vi "PH_Sequencer.panel.vi"() -> ()   [LabVIEW 2014, in "PH_Sequencer.lvlib"]
uses:
  PH_Sequencer.lvlib
  PH_Basics/PH_StatusHandler/PH_StatusHandler.GUI element.ctl
  PH_Timing/PH_Timing.Slow Trigger Settings.ctl
  PH_Timing/PH_Timing.Timing Mode.ctl
  PH_Timing/PH_Timing.Phase FEs.ctl
  PH_Sequencer.PU Information for GUI.ctl
  PH_Basics/PH_PowerUnit_BaseClass/PH_PowerUnit_BaseClass.SM States.ctl
  PH_Beamline_Chief/PH_Beamline_Chief.Section.ctl
  PH_BeamlineInformation/PH_BeamlineInformation.Powermeter.ctl
  PH_BeamlineInformation/PH_BeamlineInformation.Efficiency.ctl
  PH_Basics/PH_PP_Common/PH_PP_Common.PUs.ctl
  PH_BeamlineController/PH_BeamlineController.Source Attributes.ctl
  PH_BeamlineController/PH_BeamlineController.Sources.ctl
  PH_BeamlineController/PH_BeamlineController.Target Attributes.ctl
  PH_BeamlineController/PH_BeamlineController.Targets.ctl
  PH_BeamlineController/PH_BeamlineController.PA DP Target Attributes.ctl
  PH_BeamlineController/PH_BeamlineController.PA DP Targets.ctl
  PH_BeamlineController/PH_BeamlineController.special GUI Refs.ctl
  PH_Sequencer.Head.ctl
  PH_Sequencer.PU Information.ctl
  PH_Basics/PH_StatusHandler/PH_StatusHandler.Status.ctl
  PH_Basics/PH_SystemInformation/PH_SystemInformation.GUI Refs.ctl
  PH_BeamlineInformation/PH_BeamlineInformation.GUI Ref.ctl
  CS_Core/CSSystem/CSSystemLib/CSSystemLib.lvlib
  PH_Basics/PH_Common/PH_Common.lvlib
  PH_Timing/PH_Timing.lvlib
  PH_Beamline_Chief/PH_Beamline_Chief.lvlib
  PH_BeamlineInformation/PH_BeamlineInformation.lvlib
  PH_Basics/PH_PP_Common/PH_PP_Common.lvlib
  PH_BeamlineController/PH_BeamlineController.lvlib
  PH_Synchrolock_Watch/PH_Synchrolock_Watch.lvlib
  PH_BackreflectionMeas/PH_BackreflectionMeas.lvlib
  PH_Basics/PH_StatusHandler/PH_StatusHandler.lvlib
  PH_Basics/PH_SystemInformation/PH_SystemInformation.lvlib
  PH_Basics/PH_Class/PH_Class.lvlib
  PH_Basics/PH_PSDBWriter/PH_PSDBWriter.lvlib
  PH_Basics/PH_PowerUnit_BaseClass/PH_PowerUnit_BaseClass.lvlib
panel:
  out "PSDB Status":u32(colorbox)=6618880 caption="PSDB"
  out "Sequence length":dbl=9999.0 caption="Sequence\nlength" format="%#_4g"
  out "Shutter Exp 4 (Z6)":u32(colorbox)=6618880
  out "Shutter Exp 1":u32(colorbox)=6618880
  out "Shutter Exp 2":u32(colorbox)=6618880
  out "Shutter Exp 3":u32(colorbox)=6618880
  out "Seq SM State":string="no info"
  out "Timeout":u32(colorbox)=6618880
  out "Ready":u32(colorbox)=6618880
  out "Waiting Time":dbl=9999.0 caption="s"
  out "Status":u32(colorbox)=6618880
  out "MainAmp enabled":u32(colorbox)=6618880
  out "Emergency off":u32(colorbox)=16711680
  out "Laser enabled":u32(colorbox)=6618880
  out "PreAmp enabled":u32(colorbox)=6618880
  in  "Tab Control":T1(tab)=enum."Timing"
  in  "Remember":bool
  in  "Take Snapshot":bool caption="Force Timing"
  in  "Get PSDB Info":bool caption="Force Timing"
  out "Experiment Description":string
  in  "Shottype":i16(ring)=3 items=["experiment shot"=1, "test shot"=2, "snapshot"=3, "other"=4]
  in  "Experiment":i16(ring)=1 items=["P1"=1]
  in  "Set PSDB Settings":bool caption="Set"
  out "State PSDB":T2=2 caption="State Timing"
  out "PSDB Ready":bool
  in  "PSDB Shot Comment":string caption="Shot Comment"
  in  "Phase Frontends":T3 {"Phase" format="%#_12p"}
  in  "Timing Mode":T4 {"T2" min=0 max=6000 step=2}
  in  "Force Timing":bool
  out "State Timing":T2=2
  out "Timing Ready":bool
  in  "Slow Trigger Settings":T5
  in  "Clear Beamline":bool
  out "Beamline Ready":bool
  out "Exp LB Vacuum":bool caption="V"
  in  "PA-Backreflection-Meas":bool caption="B"
  in  "fs_Synchrolock_Watch":bool caption="S"
  in  "Accept current Path":bool caption="Accept"
  out "PA Gain":dbl=-1.0 format="%#_3g"
  out "ns_Exit_Powermeter_CurrentValue":dbl=-1.0 caption="J"
  out "fs_Nearfield_Frontend_ImageOperator_StatisticData":dbl=-1.0 caption="J"
  out "Z6 Comp Loss":dbl=-1.0 caption="Comp Loss" format="%#_3g"
  out "Z6_COS_Powermeter_CurrentValue":dbl=-1.0 caption="mJ"
  out "Z6 Conversion green":dbl=-1.0 caption="Conversion" format="%#_3g"
  out "Z6_IR_Powermeter_CurrentValue":dbl=-1.0 caption="J"
  out "Z6_green_Powermeter_CurrentValue":dbl=-1.0 caption="J"
  out "PHELIX_Beamline_LB_TB3_BL_Status":u32(colorbox)
  out "PHELIX_Beamline_PA_before_Bypass_BL_Status":u32(colorbox)
  out "PHELIX_Beamline_LL_BL_Status":u32(colorbox)
  out "PHELIX_Beamline_MA_Exit_BL_Status":u32(colorbox)
  out "PHELIX_Beamline_PA_Exit_BL_Status":u32(colorbox)
  out "PHELIX_Beamline_PA_Input_BL_Status":u32(colorbox)
  out "PHELIX_Beamline_PA_UnDelay_BL_Status":u32(colorbox)
  out "PHELIX_Beamline_fs_YLF_BL_Status":u32(colorbox)
  out "PHELIX_Beamline_YLF_BL_Status 2":u32(colorbox)
  out "PHELIX_Beamline_ns_BL_Status 2":u32(colorbox)
  out "PHELIX_Beamline_PA_Bypass_BL_Status 3":u32(colorbox)
  out "PHELIX_Beamline_PA_Bypass_BL_Status 2":u32(colorbox)
  out "PHELIX_Beamline_PA_Bypass_BL_Status 1":u32(colorbox)
  out "PHELIX_Beamline_PA_BL_Status":u32(colorbox)
  out "PHELIX_Beamline_PA_Delay_BL_Status 3":u32(colorbox)
  out "PHELIX_Beamline_PA_Delay_BL_Status 1":u32(colorbox)
  out "PHELIX_Beamline_PA_Delay_BL_Status 2":u32(colorbox)
  out "PHELIX_Beamline_MA_Z6_BL_Status":u32(colorbox)
  out "MA Gain":dbl=-1.0 format="%#_3g"
  out "PA_Exit_Powermeter_CurrentValue":dbl=-1.0 caption="J"
  out "MAS_Powermeter_CurrentValue":dbl=-1.0 caption="J"
  out "PHELIX_Beamline_LB_TB2_BL_Status":u32(colorbox)
  out "PHELIX_Beamline_MA_LB_BL_Status 2":u32(colorbox)
  out "PHELIX_Beamline_MA_LB_BL_Status 1":u32(colorbox)
  out "PHELIX_Beamline_Z6_BL_Status":u32(colorbox)
  out "PHELIX_Beamline_YLF_BL_Status 1":u32(colorbox)
  out "PHELIX_Beamline_fs_BL_Status":u32(colorbox)
  out "PHELIX_Beamline_ns_BL_Status 1":u32(colorbox)
  out "PHELIX_Beamline_PA_LL_BL_Status 2":u32(colorbox)
  out "PHELIX_Beamline_PA_LL_BL_Status 1":u32(colorbox)
  out "PHELIX_Beamline_PA_MA_BL_Status":u32(colorbox)
  out "PHELIX_Beamline_MA_LB_BL_Status 3":u32(colorbox)
  in  "Source YLF":bool caption="YLF"
  in  "Source fs-Frontend":bool caption="fs FE"
  in  "Source ns-Frontend":bool caption="ns FE"
  in  "Dump PA Delayed":bool
  in  "Dump PA Undelayed":bool
  in  "Target PreAmp":bool caption="PA"
  in  "Target Calorimeter":bool caption="MA"
  in  "Target Exp Laserbay":bool caption="Exp LB"
  in  "Target Exp Z6":bool caption="Z6"
  in  "Target Exp Laserlabor":bool caption="LL"
  in  "Target Dump Laserlabor":bool
  in  "Target Dump Z6":bool
  in  "Target Dump Laserbay":bool
  out "Beamline Z6 Ready":bool
  in  "Clear Z6 Beamline":bool
  out "PA Ready":bool=TRUE
  out "State PA Backreflection":T2=2 caption="State Timing"
  in  "Calorimeter":bool
  out "MA Ready":bool=TRUE
  out "Current Meas PA":bool caption="Current Meas\nnot linked"
  out "PP PA Ready":bool
  in  "Set Voltage PU 45mm":dbl caption="V"
  in  "PPPA_45mm_MAIN_PU":bool caption="PU 45"
  out "PU PA 45mm PILC":T6={"State"=2, "Waiting Time [s]"=1800.0, "PU State SM"=enum.".", "PU Timeout SM"=enum."."}
  out "PU PA 45mm MAIN":T6={"State"=2, "Waiting Time [s]"=1800.0, "PU State SM"=enum.".", "PU Timeout SM"=enum."."}
  in  "Set Voltage PU 19mm - 2":dbl caption="V"
  in  "PPPA_19mm_2_PU":bool caption="PU 19-2"
  out "PU PA 19mm 2":T6={"State"=2, "Waiting Time [s]"=1800.0, "PU State SM"=enum.".", "PU Timeout SM"=enum."."}
  in  "Set Voltage PU 19mm - 1":dbl caption="V"
  in  "PPPA_19mm_1_PU":bool caption="PU 19-1"
  out "PU PA 19mm 1":T6={"State"=2, "Waiting Time [s]"=1800.0, "PU State SM"=enum.".", "PU Timeout SM"=enum."."}
  in  "Set Voltage PU 45mm DP":dbl caption="V"
  in  "PPPA_45mm_DP_PU":bool caption="PU 45 DP"
  out "PU PA 45mm DP":T6={"State"=2, "Waiting Time [s]"=1800.0, "PU State SM"=enum.".", "PU Timeout SM"=enum."."}
  out "Current Voltage PU PA 19mm 1 [V]":dbl=99999.0 caption="V" format="%#_5g"
  out "Current Voltage PU PA 19mm 2 [V]":dbl=99999.0 caption="V" format="%#_5g"
  out "Current Voltage PU PA 45mm MAIN [V]":dbl=99999.0 caption="V" format="%#_5g"
  out "PP 45mm PILC in use":bool
  out "Linkage Current MA":bool caption="Current Meas\nnot linked"
  out "Linkage PPMA Rods":bool caption="Dump Rods\nnot linked"
  out "PP MA Ready":bool
  in  "Set Voltage PU 5":dbl caption="V"
  in  "PPMA_PU5":bool caption="PU 5"
  out "PU MA 5":T6={"State"=2, "Waiting Time [s]"=1800.0, "PU State SM"=enum.".", "PU Timeout SM"=enum."."}
  in  "Set Voltage PU 4":dbl caption="V"
  in  "PPMA_PU4":bool caption="PU 4"
  out "PU MA 4":T6={"State"=2, "Waiting Time [s]"=1800.0, "PU State SM"=enum.".", "PU Timeout SM"=enum."."}
  in  "Set Voltage PU 3":dbl caption="V"
  in  "PPMA_PU3":bool caption="PU 3"
  out "PU MA 3":T6={"State"=2, "Waiting Time [s]"=1800.0, "PU State SM"=enum.".", "PU Timeout SM"=enum."."}
  in  "Set Voltage PU 2":dbl caption="V"
  in  "PPMA_PU2":bool caption="PU 2"
  out "PU MA 2":T6={"State"=2, "Waiting Time [s]"=1800.0, "PU State SM"=enum.".", "PU Timeout SM"=enum."."}
  in  "Set Voltage PU 1":dbl caption="V"
  in  "PPMA_PU1":bool caption="PU 1"
  out "PU MA 1":T6={"State"=2, "Waiting Time [s]"=1800.0, "PU State SM"=enum.".", "PU Timeout SM"=enum."."}
  in  "Set Voltage FR":dbl caption="V"
  in  "PPMA_FR":bool caption="FR"
  out "PU MA FR":T6={"State"=2, "Waiting Time [s]"=1800.0, "PU State SM"=enum.".", "PU Timeout SM"=enum."."}
  out "Current Voltage PU MA 1 [V]":dbl=99999.0 caption="V" format="%#_5g"
  out "Current Voltage PU MA 2 [V]":dbl=99999.0 caption="V" format="%#_5g"
  out "Current Voltage PU MA 3 [V]":dbl=99999.0 caption="V" format="%#_5g"
  out "Current Voltage PU MA 4 [V]":dbl=99999.0 caption="V" format="%#_5g"
  out "Current Voltage PU MA 5 [V]":dbl=99999.0 caption="V" format="%#_5g"
  out "Current Voltage PU FR [V]":dbl=99999.0 caption="V" format="%#_5g"
  in  "Fire":bool
  in  "Main Off":bool
  out "error out":errorcluster
  in  "Delete":bool
  in  "error in (no error)":errorcluster
  in  "object ref":refnum<vi>
  # "PCS"
  # "3.40"
  # "s"
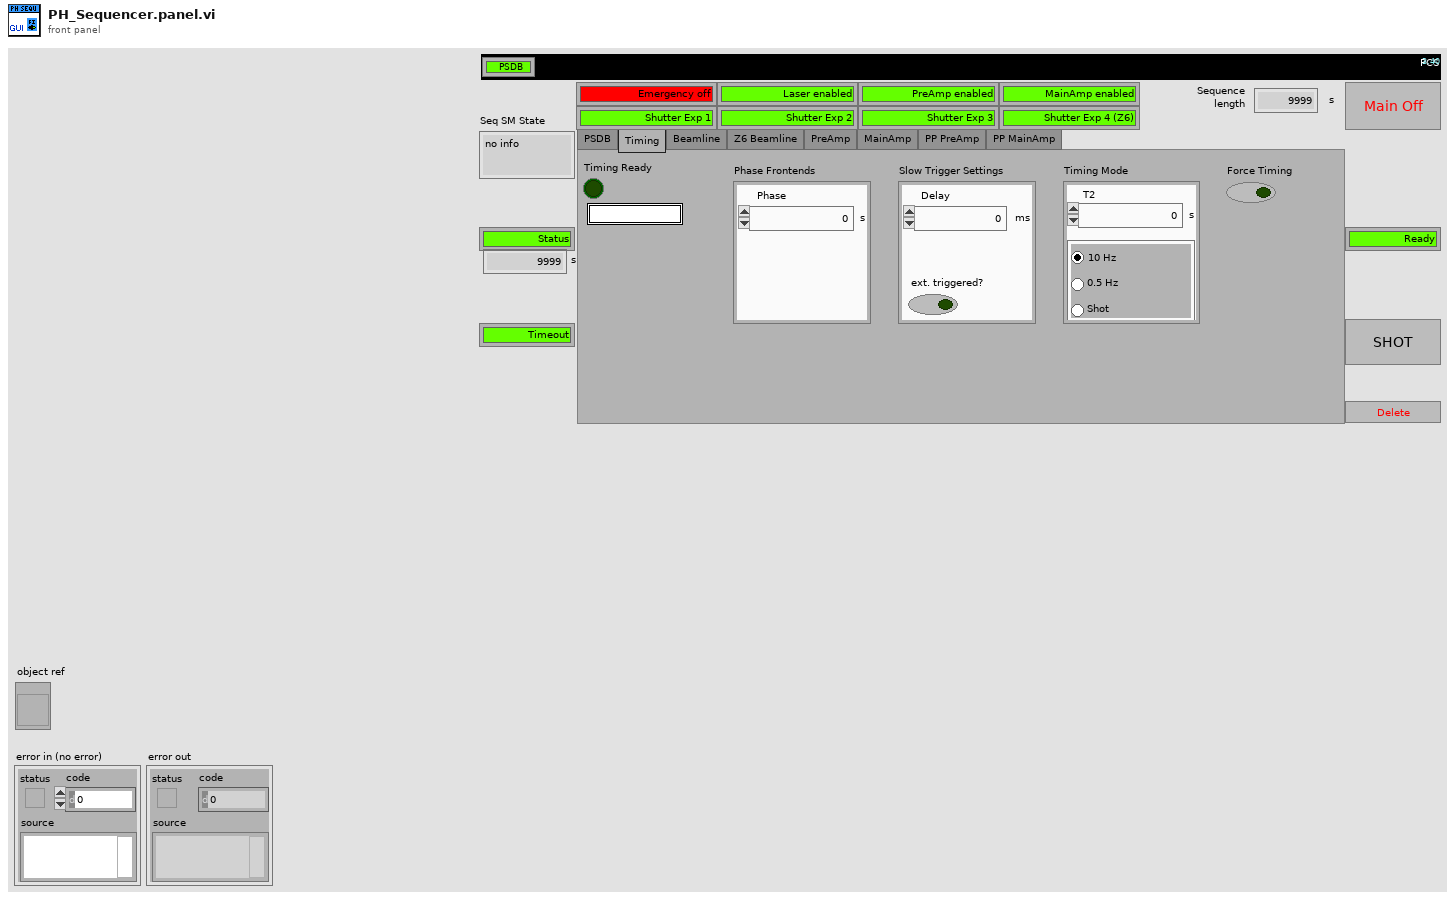
[diagram p1: front panel]
types:
  T1 = enum32{"PSDB", "Timing", "Beamline", "Z6 Beamline", "PreAmp", "MainAmp", "PP PreAmp", "PP MainAmp"}
  T2 = typedef "PH_StatusHandler.lvlib/PH_StatusHandler.GUI element.ctl" = u16
  T3 = typedef "PH_Timing.lvlib/PH_Timing.Phase FEs.ctl" = cluster{"Phase":dbl}
  T4 = typedef "PH_Timing.lvlib/PH_Timing.Timing Mode.ctl" = cluster{"T2":i16, "Modeselector":enum32{"10 Hz", "0.5 Hz", "Shot"}}
  T5 = typedef "PH_Timing.lvlib/PH_Timing.Slow Trigger Settings.ctl" = cluster{"Delay":dbl, "externally triggered?":bool}
  T6 = typedef "PH_Sequencer.lvlib/PH_Sequencer.PU Information for GUI.ctl" = cluster{"State":T2, "Waiting Time [s]":dbl, "PU State SM":T7, "PU Timeout SM":T7}
  T7 = typedef "PH_PowerUnit_BaseClass.lvlib/PH_PowerUnit_BaseClass.SM States.ctl" = enum16{".", "Stand by", "Switch PU on", "Configure", "Set Default Voltage", "Set STANDBY", "Set READY", "Wait for Shot Cmd", "Open Dump Rods", "Open Ross Relais", "Close Ross Relais", "Switch PSU on", "Switch PSU off", "Charge", "Switch GD Channel on", "Close Dump Rods", "Rods-TO", "RR-TO", "PSU-TO", "Trigger-TO"}
  T8 = typedef "PH_BeamlineController.lvlib/PH_BeamlineController.Source Attributes.ctl" = cluster{"Name":T9, "GUI Ref":refnum<vi>, "Current State":bool, "Wanted State":bool}
  T9 = typedef "PH_BeamlineController.lvlib/PH_BeamlineController.Sources.ctl" = enum16{"None", "YLF", "fs-Frontend", "ns-Frontend", "YLF and ns-Frontend", "fs- and ns-Frontend"}
  T10 = typedef "PH_BeamlineController.lvlib/PH_BeamlineController.PA DP Target Attributes.ctl" = cluster{"Name":T11, "GUI Ref":refnum<vi>, "Current State":bool, "Wanted State":bool, "Enabled":bool}
  T11 = typedef "PH_BeamlineController.lvlib/PH_BeamlineController.PA DP Targets.ctl" = enum16{"None", "Dump PA Delayed Beam", "Dump PA Undelayed Beam", "Dumps PA Delayed and Undelayed Beam"}
  T12 = typedef "PH_BeamlineController.lvlib/PH_BeamlineController.Target Attributes.ctl" = cluster{"Name":T13, "GUI Ref":refnum<vi>, "Current State":bool, "Wanted State":bool, "Enabled":bool}
  T13 = typedef "PH_BeamlineController.lvlib/PH_BeamlineController.Targets.ctl" = enum16{"None", "PreAmp", "Dump Exp Laserlab", "Exp Laserlab", "Calorimeter", "Dump Exp Laserbay", "Exp Laserbay", "Dump Exp Z6", "Exp Z6"}
  T14 = typedef "PH_BeamlineController.lvlib/PH_BeamlineController.special GUI Refs.ctl" = cluster{"PA-Backreflection-Meas":refnum<vi>, "fs_Synchrolock_Watch":refnum<vi>}
  T15 = typedef "PH_BeamlineInformation.lvlib/PH_BeamlineInformation.GUI Ref.ctl" = cluster{"BL Elements":cluster{"GUI Ref":refnum<vi>, "Beamline Section":T16}[], "Powermeters":T17, "Efficiency GUI Refs":T18, "Head GUI Refs":cluster{"PA - 19 - 1":cluster{"in Use":refnum<vi>, "voltage":refnum<vi>}, "PA - 19 - 2":cluster{"in Use":refnum<vi>, "voltage":refnum<vi>}, "PA - 45":cluster{"in Use":refnum<vi>, "voltage":refnum<vi>}, "PA - 45 - DP":cluster{"in Use":refnum<vi>, "voltage":refnum<vi>}, "MA - 1":cluster{"in Use":refnum<vi>, "voltage":refnum<vi>}, "MA - 2":cluster{"in Use":refnum<vi>, "voltage":refnum<vi>}, "MA - 3":cluster{"in Use":refnum<vi>, "voltage":refnum<vi>}, "MA - 4":cluster{"in Use":refnum<vi>, "voltage":refnum<vi>}, "MA - 5":cluster{"in Use":refnum<vi>, "voltage":refnum<vi>}, "MA - FR":cluster{"in Use":refnum<vi>, "voltage":refnum<vi>}}, "System Information GUI Refs":T19}
  T16 = typedef "PH_Beamline_Chief.lvlib/PH_Beamline_Chief.Section.ctl" = enum16{"None", "YLF", "fs", "fs-YLF", "ns", "PA-Input", "PA-Undelay", "PA-Delay", "PA-before-Bypass", "PA", "PA-Bypass", "PA-Exit", "PA-LL", "LL", "PA-MA", "MA-Exit", "MA-Z6", "Z6", "MA-LB", "LB-TB2", "LB-TB3"}
  T17 = typedef "PH_BeamlineInformation.lvlib/PH_BeamlineInformation.Powermeter.ctl" = cluster{"ns FE":cluster{"GUI Ref":refnum<vi>, "Value":dbl}, "fs FE":cluster{"GUI Ref":refnum<vi>, "Value":dbl}, "PA":cluster{"GUI Ref":refnum<vi>, "Value":dbl}, "MA":cluster{"GUI Ref":refnum<vi>, "Value":dbl}, "Z6 green":cluster{"GUI Ref":refnum<vi>, "Value":dbl}, "Z6 IR":cluster{"GUI Ref":refnum<vi>, "Value":dbl}, "Z6 COS":cluster{"GUI Ref":refnum<vi>, "Value":dbl}}
  T18 = typedef "PH_BeamlineInformation.lvlib/PH_BeamlineInformation.Efficiency.ctl" = cluster{"PA Gain":cluster{"GUI Ref":refnum<vi>, "Value":dbl}, "MA Gain":cluster{"GUI Ref":refnum<vi>, "Value":dbl}, "Z6 green Conversion":cluster{"GUI Ref":refnum<vi>, "Value":dbl}, "Z6 Comp Losses":cluster{"GUI Ref":refnum<vi>, "Value":dbl}}
  T19 = typedef "PH_SystemInformation.lvlib/PH_SystemInformation.GUI Refs.ctl" = cluster{"Laser":refnum<vi>, "PreAmp":refnum<vi>, "MainAmp":refnum<vi>, "Emergency Off":refnum<vi>, "Exp 1":refnum<vi>, "Exp 2":refnum<vi>, "Exp 3":refnum<vi>, "Exp 4":refnum<vi>, "Timing Mode GUI Ref":refnum<vi>}
  T20 = cluster{"Sources":T8[], "Side Targets":T10[], "Targets":T12[], "Experiment_VacuumControl_Experiment":refnum<vi>, "special GUI Refs":T14, "Beamline Information GUI Refs":T15}
  T21 = typedef "PH_Sequencer.lvlib/PH_Sequencer.Head.ctl" = cluster{"PowerUnit":T22, "GUI Ref":refnum<vi>, "Information":T23, "linked?":bool, "GUI Ref Current Voltage":refnum<vi>}
  T22 = typedef "PH_PP_Common.lvlib/PH_PP_Common.PUs.ctl" = enum16{"no Info", "PA-19mm-1", "PA-19mm-2", "PA-45mm-PILC", "PA-45mm-MAIN", "MA-PU-1", "MA-PU-2", "MA-PU-3", "MA-PU-4", "MA-PU-5", "MA-PU-6", "MA-FR", "MA-PILC", "PA-45mm-DP"}
  T23 = typedef "PH_Sequencer.lvlib/PH_Sequencer.PU Information.ctl" = cluster{"State":T24, "Waiting Time [s]":dbl, "PU State SM":T7, "PU Timeout SM":T7}
  T24 = typedef "PH_StatusHandler.lvlib/PH_StatusHandler.Status.ctl" = i16
  T25 = cluster{"PA - 19 - 1":cluster{"in Use":refnum<vi>, "voltage":refnum<vi>}, "PA - 19 - 2":cluster{"in Use":refnum<vi>, "voltage":refnum<vi>}, "PA - 45":cluster{"in Use":refnum<vi>, "voltage":refnum<vi>}, "PA - 45 - DP":cluster{"in Use":refnum<vi>, "voltage":refnum<vi>}, "MA - 1":cluster{"in Use":refnum<vi>, "voltage":refnum<vi>}, "MA - 2":cluster{"in Use":refnum<vi>, "voltage":refnum<vi>}, "MA - 3":cluster{"in Use":refnum<vi>, "voltage":refnum<vi>}, "MA - 4":cluster{"in Use":refnum<vi>, "voltage":refnum<vi>}, "MA - 5":cluster{"in Use":refnum<vi>, "voltage":refnum<vi>}, "MA - FR":cluster{"in Use":refnum<vi>, "voltage":refnum<vi>}}
  T26 = cluster{"GUI Ref":refnum<vi>, "Beamline Section":T16}
  T27 = typedef "PH_Sequencer.lvlib/PH_Sequencer.i attribute.ctl" = cluster{"GUI Refs":cluster{"Main Off":refnum<vi>, "Fire":refnum<vi>, "Status":refnum<vi>, "Ready":refnum<vi>, "Waiting Time":refnum<vi>, "Timeout":refnum<vi>, "PPMA Ready":refnum<vi>, "Sequencer SM State":refnum<vi>, "PPPA Ready":refnum<vi>, "Calorimeter":refnum<vi>, "Beamline Ready":refnum<vi>, "Clear Beamline":refnum<vi>, "Linkage PPMA Rods":refnum<vi>, "Linkage Current PA":refnum<vi>, "Linkage Current MA":refnum<vi>, "Timing Ready":refnum<vi>, "State Timing":refnum<vi>, "Force Timing":refnum<vi>, "PSDB Shot Comment":refnum<vi>, "State PA Backreflection":refnum<vi>, "Beamline Z6 Ready":refnum<vi>, "Clear Z6 Beamline":refnum<vi>, "Sequence length":refnum<vi>, "Timing Mode":refnum<vi>, "Slow Trigger Settings":refnum<vi>, "Experiment Description":refnum<vi>, "State PSDB":refnum<vi>, "PSDB Ready":refnum<vi>, "Set PSDB Settings":refnum<vi>, "Get PSDB Info":refnum<vi>, "Take Snapshot":refnum<vi>, "Shottype":refnum<vi>, "Experiment":refnum<vi>, "Phase Frontends":refnum<vi>, "PP 45mm PILC in use":refnum<vi>}, "Status Info":cluster{"Machine Status":T24, "WaitingTime":i32, "Timeout":bool}, "Readyness":cluster{"Ready to shot":bool, "PPMA Ready":bool, "PPPA Ready":bool, "BL Ready":bool, "Timing Ready":bool, "BL Z6 Ready":bool, "PSDBReady":bool}, "Instancenames":cluster{"PPMA Rods":string, "PP Current Meas":string, "PH Beamline Chief":string, "PA Backrefl Meas":string, "Z6 Beamline Chief":string}, "Data to read":bool, "Calorimeter":cluster{"Instancename":string, "On":bool, "linked":bool}, "Linkage":cluster{"PPMA Rods":bool, "PP Current Meas":bool, "PHELIX Beamline Chief":bool, "PA Backrefl Meas":bool, "Z6 Beamline Chief":bool}, "Timing":cluster{"Instance":string, "linked":bool, "Status":T24, "Timing Mode":T4, "Slow Trigger Settings":T5, "Info available":cluster{"ext SlowTrigger":bool, "T2":bool, "Mode":bool, "Delay Slow Trigger":bool, "Phase FEs":bool}, "FE Phase":T3}, "Service ID R2S":i32, "PSDB":cluster{"Controller Instance":string, "Controller Status":T24, "Controller linked":bool, "Settings acknowledged":bool, "Current Experiment ID":i16, "Current Shot Type":i16, "Current Comment":string, "Remember Settings":bool, "Write 2 early":bool}, "PSDB Data":cluster{"Main Off?":bool, "Sequence Length":dbl, "Sequence startet":timestamp}, "6P 4Q Positions":cluster{"Instancename":string, "linked":bool, "Position":T28}[], "PUs":T21[]}
  T28 = typedef "PH_4_Pos_Selector.lvlib/PH_4_Pos_Selector.Position Selector.ctl" = u16
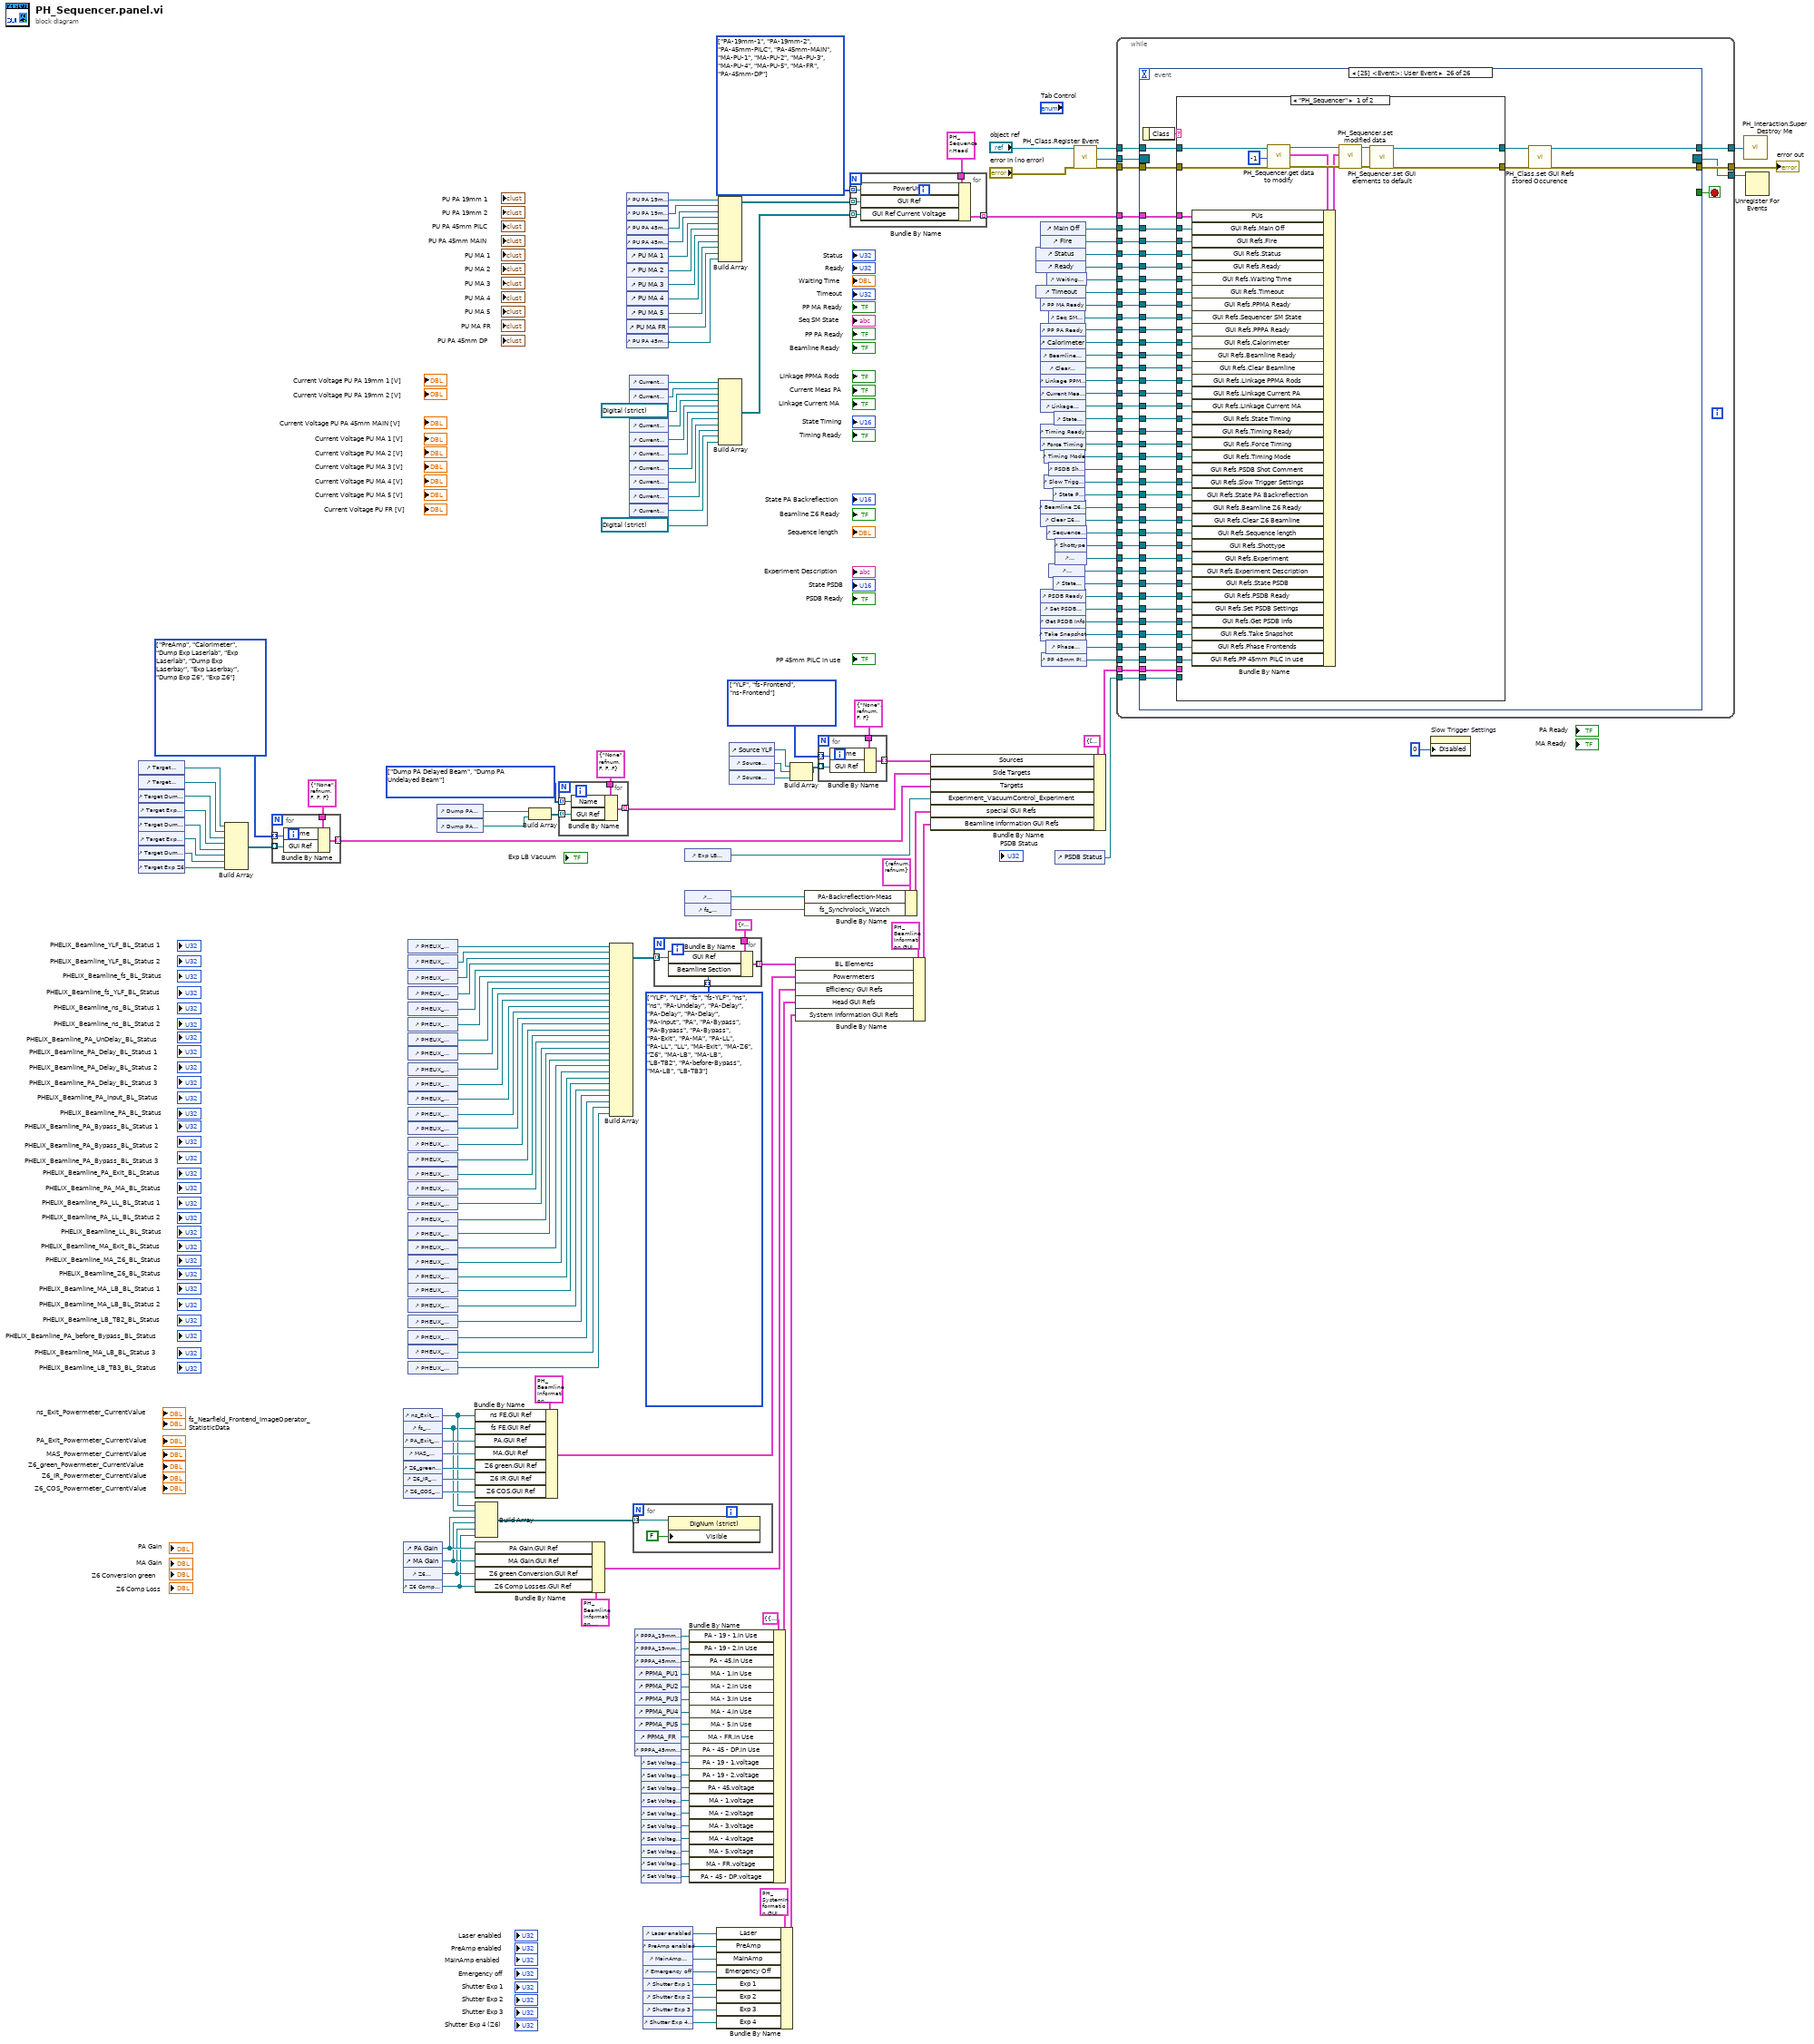
[diagram p0: block diagram]
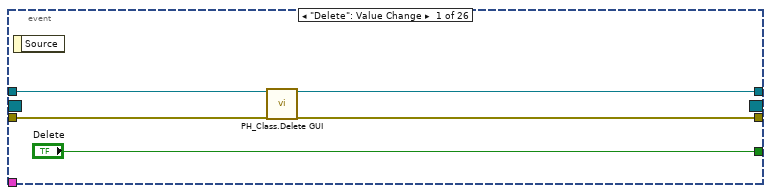
[diagram p2: hidden frame]
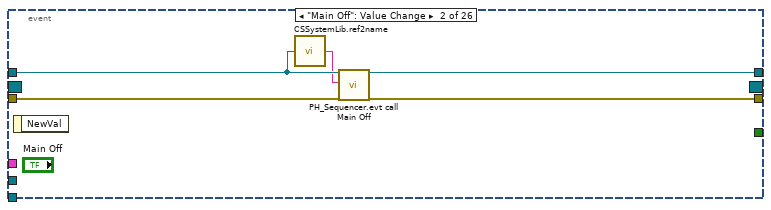
[diagram p3: hidden frame]
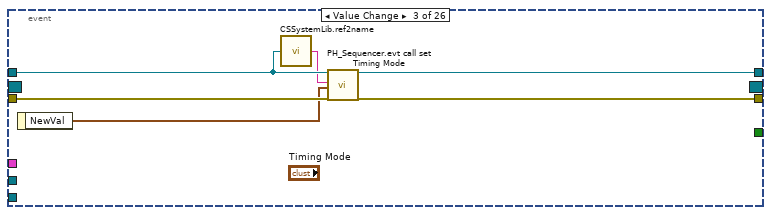
[diagram p4: hidden frame]
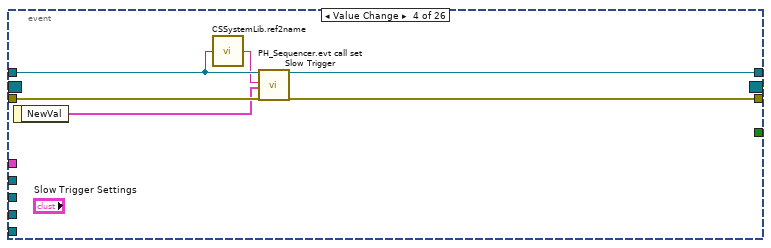
[diagram p5: hidden frame]
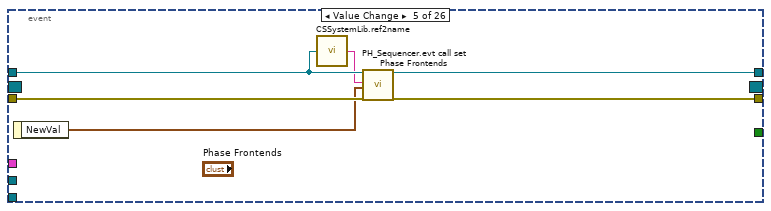
[diagram p6: hidden frame]
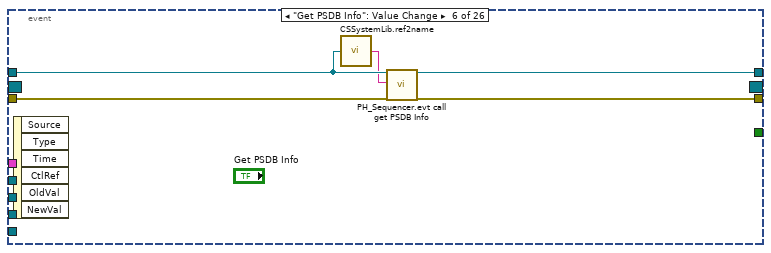
[diagram p7: hidden frame]
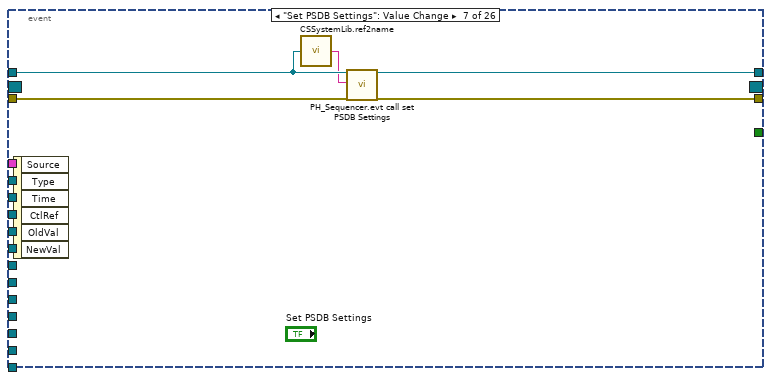
[diagram p8: hidden frame]
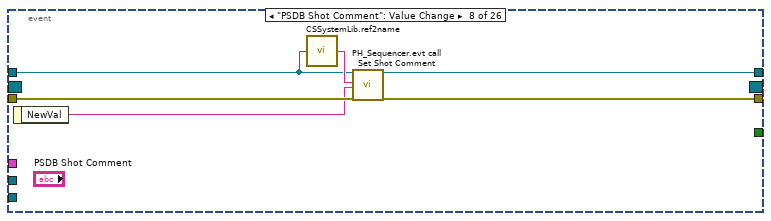
[diagram p9: hidden frame]
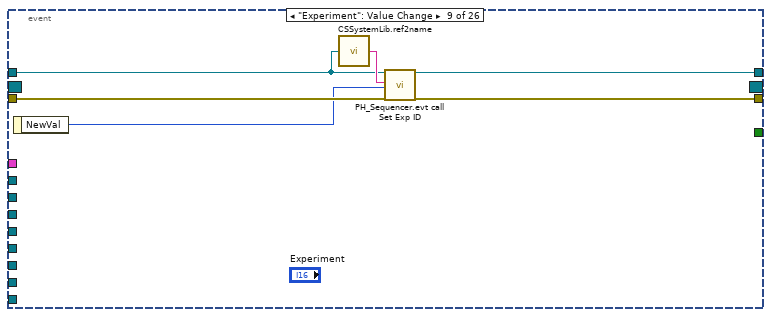
[diagram p10: hidden frame]
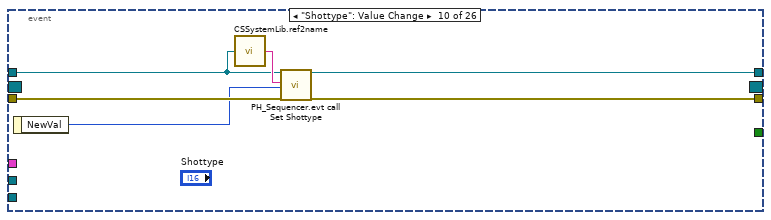
[diagram p11: hidden frame]
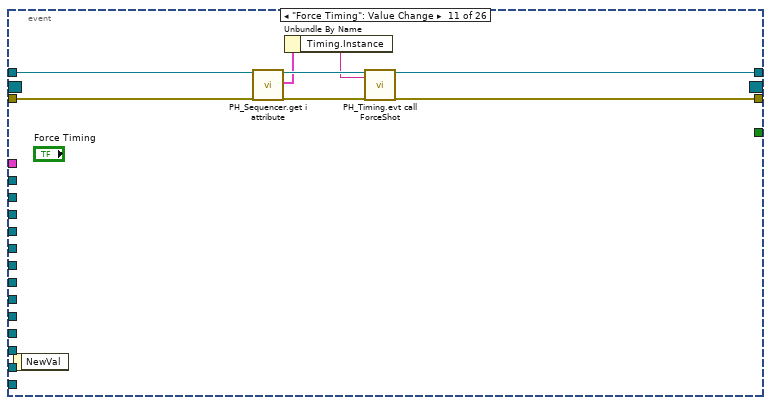
[diagram p12: hidden frame]
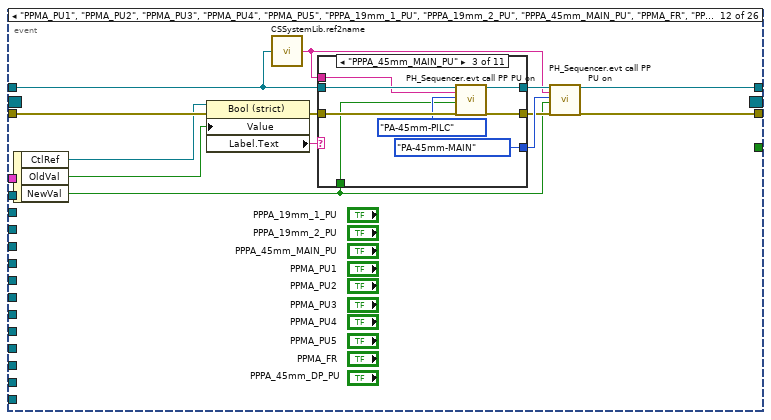
[diagram p13: hidden frame]
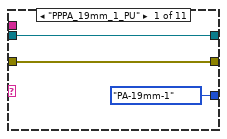
[diagram p14: hidden frame]
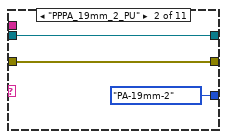
[diagram p15: hidden frame]
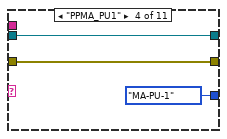
[diagram p16: hidden frame]
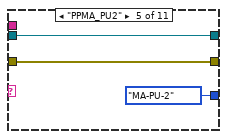
[diagram p17: hidden frame]
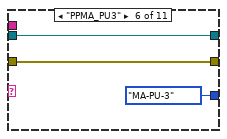
[diagram p18: hidden frame]
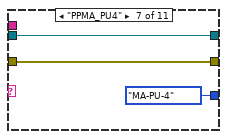
[diagram p19: hidden frame]
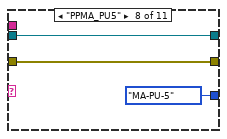
[diagram p20: hidden frame]
diagram:
  w78 = T11[] [enum."Dump PA Delayed Beam", enum."Dump PA Undelayed Beam"] items=["None", "Dump PA Delayed Beam", "Dump PA Undelayed Beam", "Dumps PA Delayed and Undelayed Beam"]
  w98 = T13[] [enum."PreAmp", enum."Calorimeter", enum."Dump Exp Laserlab", enum."Exp Laserlab", enum."Dump Exp Laserbay", enum."Exp Laserbay", enum."Dump Exp Z6", enum."Exp Z6"] items=["None", "PreAmp", "Dump Exp Laserlab", "Exp Laserlab", "Calorimeter", "Dump Exp Laserbay", "Exp Laserbay", "Dump Exp Z6", "Exp Z6"]
  w102 = T9[] [enum."YLF", enum."fs-Frontend", enum."ns-Frontend"] items=["None", "YLF", "fs-Frontend", "ns-Frontend", "YLF and ns-Frontend", "fs- and ns-Frontend"]
  w108 = T22[] [enum."PA-19mm-1", enum."PA-19mm-2", enum."PA-45mm-PILC", enum."PA-45mm-MAIN", enum."MA-PU-1", enum."MA-PU-2", enum."MA-PU-3", enum."MA-PU-4", enum."MA-PU-5", enum."MA-FR", enum."PA-45mm-DP"] items=["no Info", "PA-19mm-1", "PA-19mm-2", "PA-45mm-PILC", "PA-45mm-MAIN", "MA-PU-1", "MA-PU-2", "MA-PU-3", "MA-PU-4", "MA-PU-5", "MA-PU-6", "MA-FR", "MA-PILC", "PA-45mm-DP"]
  w145 = T16[] [enum."YLF", enum."YLF", enum."fs", enum."fs-YLF", enum."ns", enum."ns", enum."PA-Undelay", enum."PA-Delay", enum."PA-Delay", enum."PA-Delay", enum."PA-Input", enum."PA", enum."PA-Bypass", enum."PA-Bypass", enum."PA-Bypass", enum."PA-Exit", enum."PA-MA", enum."PA-LL", enum."PA-LL", enum."LL", enum."MA-Exit", enum."MA-Z6", enum."Z6", enum."MA-LB", enum."MA-LB", enum."LB-TB2", enum."PA-before-Bypass", enum."MA-LB", enum."LB-TB3"] items=["None", "YLF", "fs", "fs-YLF", "ns", "PA-Input", "PA-Undelay", "PA-Delay", "PA-before-Bypass", "PA", "PA-Bypass", "PA-Exit", "PA-LL", "LL", "PA-MA", "MA-Exit", "MA-Z6", "Z6", "MA-LB", "LB-TB2", "LB-TB3"]
  n1 = control-ref of="Target PreAmp"() -> (w91:refnum<vi>)
  n2 = control-ref of="Target Calorimeter"() -> (w90:refnum<vi>)
  n3 = control-ref of="Target Dump Laserlabor"() -> (w89:refnum<vi>)
  n4 = control-ref of="Target Exp Laserlabor"() -> (w88:refnum<vi>)
  n5 = control-ref of="Target Dump Laserbay"() -> (w87:refnum<vi>)
  n6 = control-ref of="Target Exp Laserbay"() -> (w86:refnum<vi>)
  n7 = control-ref of="Target Dump Z6"() -> (w85:refnum<vi>)
  n8 = control-ref of="Target Exp Z6"() -> (w84:refnum<vi>)
  n9 = Build Array(w91, w90, w89, w88, w87, w86, w85, w84) -> (w99:refnum<vi>[])
  n10 = for {
    tunnel: T12 {"Name"=enum."None", "GUI Ref"=refnum, "Current State"=FALSE, "Wanted State"=FALSE, "Enabled"=FALSE} ("Target Attributes") -> [w191]
    tunnel: [w190] -> w71 mode=indexing
    tunnel: w98 -> [w189] mode=indexing
    tunnel: w99 -> [w188] mode=indexing
    n11 = Bundle By Name(cluster=w191, "Name"=w189, "GUI Ref"=w188) -> (w190:T12)
  }
  n12 = control-ref of="ns_Exit_Powermeter_CurrentValue"() -> (w137:refnum<vi>)
  n13 = control-ref of="fs_Nearfield_Frontend_ImageOperator_StatisticData"() -> (w136:refnum<vi>)
  n14 = control-ref of="PA_Exit_Powermeter_CurrentValue"() -> (w142:refnum<vi>)
  n15 = control-ref of="MAS_Powermeter_CurrentValue"() -> (w141:refnum<vi>)
  n16 = control-ref of="Z6_green_Powermeter_CurrentValue"() -> (w140:refnum<vi>)
  n17 = control-ref of="Z6_IR_Powermeter_CurrentValue"() -> (w139:refnum<vi>)
  n18 = control-ref of="Z6_COS_Powermeter_CurrentValue"() -> (w138:refnum<vi>)
  n19 = control-ref of="PA Gain"() -> (w135:refnum<vi>)
  n20 = control-ref of="MA Gain"() -> (w133:refnum<vi>)
  n21 = control-ref of="Z6 Conversion green"() -> (w132:refnum<vi>)
  n22 = control-ref of="Z6 Comp Loss"() -> (w131:refnum<vi>)
  n23 = control-ref of="PHELIX_Beamline_YLF_BL_Status 1"() -> (w184:refnum<vi>)
  n24 = control-ref of="PHELIX_Beamline_YLF_BL_Status 2"() -> (w183:refnum<vi>)
  n25 = control-ref of="PHELIX_Beamline_fs_BL_Status"() -> (w182:refnum<vi>)
  n26 = control-ref of="PHELIX_Beamline_fs_YLF_BL_Status"() -> (w181:refnum<vi>)
  n27 = control-ref of="PHELIX_Beamline_ns_BL_Status 1"() -> (w180:refnum<vi>)
  n28 = control-ref of="PHELIX_Beamline_ns_BL_Status 2"() -> (w179:refnum<vi>)
  n29 = control-ref of="PHELIX_Beamline_PA_UnDelay_BL_Status"() -> (w166:refnum<vi>)
  n30 = control-ref of="PHELIX_Beamline_PA_Delay_BL_Status 1"() -> (w165:refnum<vi>)
  n31 = control-ref of="PHELIX_Beamline_PA_Delay_BL_Status 2"() -> (w164:refnum<vi>)
  n32 = control-ref of="PHELIX_Beamline_PA_Delay_BL_Status 3"() -> (w163:refnum<vi>)
  n33 = control-ref of="PHELIX_Beamline_PA_Input_BL_Status"() -> (w178:refnum<vi>)
  n34 = control-ref of="PHELIX_Beamline_PA_BL_Status"() -> (w162:refnum<vi>)
  n35 = control-ref of="PHELIX_Beamline_PA_Bypass_BL_Status 1"() -> (w161:refnum<vi>)
  n36 = control-ref of="PHELIX_Beamline_PA_Bypass_BL_Status 2"() -> (w160:refnum<vi>)
  n37 = control-ref of="PHELIX_Beamline_PA_Bypass_BL_Status 3"() -> (w159:refnum<vi>)
  n38 = control-ref of="PHELIX_Beamline_PA_Exit_BL_Status"() -> (w177:refnum<vi>)
  n39 = control-ref of="PHELIX_Beamline_PA_MA_BL_Status"() -> (w176:refnum<vi>)
  n40 = control-ref of="PHELIX_Beamline_PA_LL_BL_Status 1"() -> (w175:refnum<vi>)
  n41 = control-ref of="PHELIX_Beamline_PA_LL_BL_Status 2"() -> (w174:refnum<vi>)
  n42 = control-ref of="PHELIX_Beamline_LL_BL_Status"() -> (w173:refnum<vi>)
  n43 = control-ref of="PHELIX_Beamline_MA_Exit_BL_Status"() -> (w172:refnum<vi>)
  n44 = control-ref of="PHELIX_Beamline_MA_Z6_BL_Status"() -> (w167:refnum<vi>)
  n45 = control-ref of="PHELIX_Beamline_Z6_BL_Status"() -> (w171:refnum<vi>)
  n46 = control-ref of="PHELIX_Beamline_MA_LB_BL_Status 1"() -> (w170:refnum<vi>)
  n47 = control-ref of="PHELIX_Beamline_MA_LB_BL_Status 2"() -> (w169:refnum<vi>)
  n48 = control-ref of="PHELIX_Beamline_LB_TB2_BL_Status"() -> (w168:refnum<vi>)
  n49 = control-ref of="PHELIX_Beamline_PA_before_Bypass_BL_Status"() -> (w158:refnum<vi>)
  n50 = control-ref of="PHELIX_Beamline_MA_LB_BL_Status 3"() -> (w149:refnum<vi>)
  n51 = control-ref of="PHELIX_Beamline_LB_TB3_BL_Status"() -> (w148:refnum<vi>)
  n52 = control-ref of="Dump PA Delayed"() -> (w92:refnum<vi>)
  n53 = control-ref of="Dump PA Undelayed"() -> (w79:refnum<vi>)
  n54 = Bundle By Name(cluster=T17 {"ns FE"={"GUI Ref"=refnum, "Value"=-1.0}, "fs FE"={"GUI Ref"=refnum, "Value"=-1.0}, "PA"={"GUI Ref"=refnum, "Value"=-1.0}, "MA"={"GUI Ref"=refnum, "Value"=-1.0}, "Z6 green"={"GUI Ref"=refnum, "Value"=-1.0}, "Z6 IR"={"GUI Ref"=refnum, "Value"=-1.0}, "Z6 COS"={"GUI Ref"=refnum, "Value"=-1.0}} ("Powermeters"), "ns FE.GUI Ref"=w137, "fs FE.GUI Ref"=w136, "PA.GUI Ref"=w142, "MA.GUI Ref"=w141, "Z6 green.GUI Ref"=w140, "Z6 IR.GUI Ref"=w139, "Z6 COS.GUI Ref"=w138) -> (w106:T17)
  n55 = Build Array(w137, w136, w135, w133, w132, w131) -> (w134:refnum<vi>[])
  n56 = Bundle By Name(cluster=T18 {"PA Gain"={"GUI Ref"=refnum, "Value"=-1.0}, "MA Gain"={"GUI Ref"=refnum, "Value"=-1.0}, "Z6 green Conversion"={"GUI Ref"=refnum, "Value"=-1.0}, "Z6 Comp Losses"={"GUI Ref"=refnum, "Value"=-1.0}} ("Efficiency GUI Refs"), "PA Gain.GUI Ref"=w135, "MA Gain.GUI Ref"=w133, "Z6 green Conversion.GUI Ref"=w132, "Z6 Comp Losses.GUI Ref"=w131) -> (w105:T18)
  n57 = Build Array(w92, w79) -> (w96:refnum<vi>[])
  n58 = for {
    tunnel: T10 {"Name"=enum."None", "GUI Ref"=refnum, "Current State"=FALSE, "Wanted State"=FALSE, "Enabled"=FALSE} ("Target") -> [w195]
    tunnel: [w194] -> w72 mode=indexing
    tunnel: w78 -> [w193] mode=indexing
    tunnel: w96 -> [w192] mode=indexing
    n59 = Bundle By Name(cluster=w195, "Name"=w193, "GUI Ref"=w192) -> (w194:T10)
  }
  n60 = Build Array(w184, w183, w182, w181, w180, w179, w166, w165, w164, w163, w178, w162, w161, w160, w159, w177, w176, w175, w174, w173, w172, w167, w171, w170, w169, w168, w158, w149, w148) -> (w146:refnum<vi>[])
  n61 = control-ref of="PU PA 19mm 1"() -> (w14:refnum<vi>)
  n62 = control-ref of="PU PA 19mm 2"() -> (w13:refnum<vi>)
  n63 = control-ref of="PU PA 45mm PILC"() -> (w12:refnum<vi>)
  n64 = control-ref of="PU PA 45mm MAIN"() -> (w11:refnum<vi>)
  n65 = control-ref of="PU MA 1"() -> (w10:refnum<vi>)
  n66 = control-ref of="PU MA 2"() -> (w9:refnum<vi>)
  n67 = control-ref of="PU MA 3"() -> (w8:refnum<vi>)
  n68 = control-ref of="PU MA 4"() -> (w7:refnum<vi>)
  n69 = control-ref of="PU MA 5"() -> (w6:refnum<vi>)
  n70 = control-ref of="PU MA FR"() -> (w5:refnum<vi>)
  n71 = control-ref of="PU PA 45mm DP"() -> (w4:refnum<vi>)
  n72 = control-ref of="Current Voltage PU PA 19mm 1 [V]"() -> (w26:refnum<vi>)
  n73 = control-ref of="Current Voltage PU PA 19mm 2 [V]"() -> (w25:refnum<vi>)
  n74 = control-ref of="Current Voltage PU PA 45mm MAIN [V]"() -> (w23:refnum<vi>)
  n75 = control-ref of="Current Voltage PU MA 1 [V]"() -> (w22:refnum<vi>)
  n76 = control-ref of="Current Voltage PU MA 2 [V]"() -> (w21:refnum<vi>)
  n77 = control-ref of="Current Voltage PU MA 3 [V]"() -> (w20:refnum<vi>)
  n78 = control-ref of="Current Voltage PU MA 4 [V]"() -> (w19:refnum<vi>)
  n79 = control-ref of="Current Voltage PU MA 5 [V]"() -> (w18:refnum<vi>)
  n80 = control-ref of="Current Voltage PU FR [V]"() -> (w17:refnum<vi>)
  n81 = for {
    tunnel: w134 -> [w197] mode=indexing
    n82 = property class="DigNum (strict)"(reference=w197, "Visible"=FALSE) -> ()  [unwired: 1 in, 2 out]
  }
  n83 = control-ref of="PPPA_19mm_1_PU"() -> (w130:refnum<vi>)
  n84 = control-ref of="PPPA_19mm_2_PU"() -> (w129:refnum<vi>)
  n85 = control-ref of="PPPA_45mm_MAIN_PU"() -> (w128:refnum<vi>)
  n86 = control-ref of="PPMA_PU1"() -> (w127:refnum<vi>)
  n87 = control-ref of="PPMA_PU2"() -> (w126:refnum<vi>)
  n88 = control-ref of="PPMA_PU3"() -> (w125:refnum<vi>)
  n89 = control-ref of="PPMA_PU4"() -> (w124:refnum<vi>)
  n90 = control-ref of="PPMA_PU5"() -> (w123:refnum<vi>)
  n91 = control-ref of="PPMA_FR"() -> (w122:refnum<vi>)
  n92 = control-ref of="PPPA_45mm_DP_PU"() -> (w110:refnum<vi>)
  n93 = control-ref of="Set Voltage PU 19mm - 1"() -> (w119:refnum<vi>)
  n94 = control-ref of="Set Voltage PU 19mm - 2"() -> (w118:refnum<vi>)
  n95 = control-ref of="Set Voltage PU 45mm"() -> (w117:refnum<vi>)
  n96 = control-ref of="Set Voltage PU 1"() -> (w116:refnum<vi>)
  n97 = control-ref of="Set Voltage PU 2"() -> (w115:refnum<vi>)
  n98 = control-ref of="Set Voltage PU 3"() -> (w114:refnum<vi>)
  n99 = control-ref of="Set Voltage PU 4"() -> (w113:refnum<vi>)
  n100 = control-ref of="Set Voltage PU 5"() -> (w112:refnum<vi>)
  n101 = control-ref of="Set Voltage FR"() -> (w111:refnum<vi>)
  n102 = control-ref of="Set Voltage PU 45mm DP"() -> (w109:refnum<vi>)
  n103 = control-ref of="Laser enabled"() -> (w157:refnum<vi>)
  n104 = control-ref of="PreAmp enabled"() -> (w156:refnum<vi>)
  n105 = control-ref of="MainAmp enabled"() -> (w155:refnum<vi>)
  n106 = control-ref of="Emergency off"() -> (w154:refnum<vi>)
  n107 = control-ref of="Shutter Exp 1"() -> (w153:refnum<vi>)
  n108 = control-ref of="Shutter Exp 2"() -> (w152:refnum<vi>)
  n109 = control-ref of="Shutter Exp 3"() -> (w151:refnum<vi>)
  n110 = control-ref of="Shutter Exp 4 (Z6)"() -> (w150:refnum<vi>)
  n111 = for {
    tunnel: T26 {"GUI Ref"=refnum, "Beamline Section"=enum."None"} ("BL Element") -> [w201]
    tunnel: [w200] -> w107 mode=indexing
    tunnel: w146 -> [w199] mode=indexing
    tunnel: w145 -> [w198] mode=indexing
    n112 = Bundle By Name(cluster=w201, "GUI Ref"=w199, "Beamline Section"=w198) -> (w200:T26)
  }
  n113 = control-ref of="Exp LB Vacuum"() -> (w70:refnum<vi>)
  n114 = control-ref of="PA-Backreflection-Meas"() -> (w82:refnum<vi>)
  n115 = control-ref of="fs_Synchrolock_Watch"() -> (w81:refnum<vi>)
  n116 = Bundle By Name(cluster=T25 {"PA - 19 - 1"={"in Use"=refnum, "voltage"=refnum}, "PA - 19 - 2"={"in Use"=refnum, "voltage"=refnum}, "PA - 45"={"in Use"=refnum, "voltage"=refnum}, "PA - 45 - DP"={"in Use"=refnum, "voltage"=refnum}, "MA - 1"={"in Use"=refnum, "voltage"=refnum}, "MA - 2"={"in Use"=refnum, "voltage"=refnum}, "MA - 3"={"in Use"=refnum, "voltage"=refnum}, "MA - 4"={"in Use"=refnum, "voltage"=refnum}, "MA - 5"={"in Use"=refnum, "voltage"=refnum}, "MA - FR"={"in Use"=refnum, "voltage"=refnum}} ("Head GUI Refs"), "PA - 19 - 1.in Use"=w130, "PA - 19 - 2.in Use"=w129, "PA - 45.in Use"=w128, "MA - 1.in Use"=w127, "MA - 2.in Use"=w126, "MA - 3.in Use"=w125, "MA - 4.in Use"=w124, "MA - 5.in Use"=w123, "MA - FR.in Use"=w122, "PA - 45 - DP.in Use"=w110, "PA - 19 - 1.voltage"=w119, "PA - 19 - 2.voltage"=w118, "PA - 45.voltage"=w117, "MA - 1.voltage"=w116, "MA - 2.voltage"=w115, "MA - 3.voltage"=w114, "MA - 4.voltage"=w113, "MA - 5.voltage"=w112, "MA - FR.voltage"=w111, "PA - 45 - DP.voltage"=w109) -> (w104:T25)
  n117 = Bundle By Name(cluster=T19 {"Laser"=refnum, "PreAmp"=refnum, "MainAmp"=refnum, "Emergency Off"=refnum, "Exp 1"=refnum, "Exp 2"=refnum, "Exp 3"=refnum, "Exp 4"=refnum, "Timing Mode GUI Ref"=refnum} ("Input for System Information"), "Laser"=w157, "PreAmp"=w156, "MainAmp"=w155, "Emergency Off"=w154, "Exp 1"=w153, "Exp 2"=w152, "Exp 3"=w151, "Exp 4"=w150) -> (w75:T19)
  n118 = Build Array(w14, w13, w12, w11, w10, w9, w8, w7, w6, w5, w4) -> (w121:refnum<vi>[])
  n119 = Build Array(w26, w25, refnum<vi> refnum ("element"), w23, w22, w21, w20, w19, w18, w17, refnum<vi> refnum ("element")) -> (w15:refnum<vi>[])
  n120 = control-ref of="Source YLF"() -> (w95:refnum<vi>)
  n121 = control-ref of="Source fs-Frontend"() -> (w94:refnum<vi>)
  n122 = control-ref of="Source ns-Frontend"() -> (w93:refnum<vi>)
  n123 = Build Array(w95, w94, w93) -> (w101:refnum<vi>[])
  n124 = Bundle By Name(cluster=T15 {"BL Elements"=[], "Powermeters"={"ns FE"={"GUI Ref"=refnum, "Value"=-1.0}, "fs FE"={"GUI Ref"=refnum, "Value"=-1.0}, "PA"={"GUI Ref"=refnum, "Value"=-1.0}, "MA"={"GUI Ref"=refnum, "Value"=-1.0}, "Z6 green"={"GUI Ref"=refnum, "Value"=-1.0}, "Z6 IR"={"GUI Ref"=refnum, "Value"=-1.0}, "Z6 COS"={"GUI Ref"=refnum, "Value"=-1.0}}, "Efficiency GUI Refs"={"PA Gain"={"GUI Ref"=refnum, "Value"=-1.0}, "MA Gain"={"GUI Ref"=refnum, "Value"=-1.0}, "Z6 green Conversion"={"GUI Ref"=refnum, "Value"=-1.0}, "Z6 Comp Losses"={"GUI Ref"=refnum, "Value"=-1.0}}, "Head GUI Refs"={"PA - 19 - 1"={"in Use"=refnum, "voltage"=refnum}, "PA - 19 - 2"={"in Use"=refnum, "voltage"=refnum}, "PA - 45"={"in Use"=refnum, "voltage"=refnum}, "PA - 45 - DP"={"in Use"=refnum, "voltage"=refnum}, "MA - 1"={"in Use"=refnum, "voltage"=refnum}, "MA - 2"={"in Use"=refnum, "voltage"=refnum}, "MA - 3"={"in Use"=refnum, "voltage"=refnum}, "MA - 4"={"in Use"=refnum, "voltage"=refnum}, "MA - 5"={"in Use"=refnum, "voltage"=refnum}, "MA - FR"={"in Use"=refnum, "voltage"=refnum}}, "System Information GUI Refs"={"Laser"=refnum, "PreAmp"=refnum, "MainAmp"=refnum, "Emergency Off"=refnum, "Exp 1"=refnum, "Exp 2"=refnum, "Exp 3"=refnum, "Exp 4"=refnum, "Timing Mode GUI Ref"=refnum}} ("BeamlineInformation GUI Refs"), "BL Elements"=w107, "Powermeters"=w106, "Efficiency GUI Refs"=w105, "Head GUI Refs"=w104, "System Information GUI Refs"=w75) -> (w68:T15)
  n125 = Bundle By Name(cluster=T14 {"PA-Backreflection-Meas"=refnum, "fs_Synchrolock_Watch"=refnum} ("GUI Refs"), "PA-Backreflection-Meas"=w82, "fs_Synchrolock_Watch"=w81) -> (w69:T14)
  n126 = for {
    tunnel: T8 {"Name"=enum."None", "GUI Ref"=refnum, "Current State"=FALSE, "Wanted State"=FALSE} ("Source Attributes") -> [w205]
    tunnel: [w204] -> w73 mode=indexing
    tunnel: w102 -> [w203] mode=indexing
    tunnel: w101 -> [w202] mode=indexing
    n127 = Bundle By Name(cluster=w205, "Name"=w203, "GUI Ref"=w202) -> (w204:T8)
  }
  n128 = for {
    tunnel: w121 -> [w208] mode=indexing
    tunnel: w108 -> [w207] mode=indexing
    tunnel: [w210] -> w59 mode=indexing
    tunnel: T21 {"PowerUnit"=enum."no Info", "GUI Ref"=refnum, "Information"={"State"=0, "Waiting Time [s]"=0.0, "PU State SM"=enum.".", "PU Timeout SM"=enum."."}, "linked?"=FALSE, "GUI Ref Current Voltage"=refnum} ("Head") -> [w209]
    tunnel: w15 -> [w206] mode=indexing
    n129 = Bundle By Name(cluster=w209, "PowerUnit"=w207, "GUI Ref"=w208, "GUI Ref Current Voltage"=w206) -> (w210:T21)
  }
  n130 = Bundle By Name(cluster=T20 {"Sources"=[], "Side Targets"=[], "Targets"=[], "Experiment_VacuumControl_Experiment"=refnum, "special GUI Refs"={"PA-Backreflection-Meas"=refnum, "fs_Synchrolock_Watch"=refnum}, "Beamline Information GUI Refs"={"BL Elements"=[], "Powermeters"={"ns FE"={"GUI Ref"=refnum, "Value"=-1.0}, "fs FE"={"GUI Ref"=refnum, "Value"=-1.0}, "PA"={"GUI Ref"=refnum, "Value"=-1.0}, "MA"={"GUI Ref"=refnum, "Value"=-1.0}, "Z6 green"={"GUI Ref"=refnum, "Value"=-1.0}, "Z6 IR"={"GUI Ref"=refnum, "Value"=-1.0}, "Z6 COS"={"GUI Ref"=refnum, "Value"=-1.0}}, "Efficiency GUI Refs"={"PA Gain"={"GUI Ref"=refnum, "Value"=-1.0}, "MA Gain"={"GUI Ref"=refnum, "Value"=-1.0}, "Z6 green Conversion"={"GUI Ref"=refnum, "Value"=-1.0}, "Z6 Comp Losses"={"GUI Ref"=refnum, "Value"=-1.0}}, "Head GUI Refs"={"PA - 19 - 1"={"in Use"=refnum, "voltage"=refnum}, "PA - 19 - 2"={"in Use"=refnum, "voltage"=refnum}, "PA - 45"={"in Use"=refnum, "voltage"=refnum}, "PA - 45 - DP"={"in Use"=refnum, "voltage"=refnum}, "MA - 1"={"in Use"=refnum, "voltage"=refnum}, "MA - 2"={"in Use"=refnum, "voltage"=refnum}, "MA - 3"={"in Use"=refnum, "voltage"=refnum}, "MA - 4"={"in Use"=refnum, "voltage"=refnum}, "MA - 5"={"in Use"=refnum, "voltage"=refnum}, "MA - FR"={"in Use"=refnum, "voltage"=refnum}}, "System Information GUI Refs"={"Laser"=refnum, "PreAmp"=refnum, "MainAmp"=refnum, "Emergency Off"=refnum, "Exp 1"=refnum, "Exp 2"=refnum, "Exp 3"=refnum, "Exp 4"=refnum, "Timing Mode GUI Ref"=refnum}}} ("Beamline Controller GUI Refs"), "Sources"=w73, "Side Targets"=w72, "Targets"=w71, "Experiment_VacuumControl_Experiment"=w70, "special GUI Refs"=w69, "Beamline Information GUI Refs"=w68) -> (w63:T20)
  n131 = control-ref of="Status"() -> (w56:refnum<vi>)
  n132 = control-ref of="Ready"() -> (w55:refnum<vi>)
  n133 = control-ref of="Timeout"() -> (w53:refnum<vi>)
  n134 = control-ref of="Main Off"() -> (w58:refnum<vi>)
  n135 = control-ref of="Fire"() -> (w57:refnum<vi>)
  n136 = control-ref of="PP MA Ready"() -> (w52:refnum<vi>)
  n137 = control-ref of="PP PA Ready"() -> (w50:refnum<vi>)
  n138 = control-ref of="Calorimeter"() -> (w49:refnum<vi>)
  n139 = control-ref of="Beamline Ready"() -> (w48:refnum<vi>)
  n140 = control-ref of="Clear Beamline"() -> (w47:refnum<vi>)
  n141 = control-ref of="Linkage PPMA Rods"() -> (w46:refnum<vi>)
  n142 = control-ref of="Current Meas PA"() -> (w45:refnum<vi>)
  n143 = control-ref of="Linkage Current MA"() -> (w44:refnum<vi>)
  n144 = control-ref of="Timing Ready"() -> (w43:refnum<vi>)
  n145 = control-ref of="Force Timing"() -> (w42:refnum<vi>)
  n146 = control-ref of="Beamline Z6 Ready"() -> (w38:refnum<vi>)
  n147 = control-ref of="Clear Z6 Beamline"() -> (w37:refnum<vi>)
  n148 = control-ref of="PSDB Ready"() -> (w32:refnum<vi>)
  n149 = control-ref of="Set PSDB Settings"() -> (w31:refnum<vi>)
  n150 = control-ref of="Get PSDB Info"() -> (w30:refnum<vi>)
  n151 = control-ref of="Take Snapshot"() -> (w29:refnum<vi>)
  n152 = control-ref of="PP 45mm PILC in use"() -> (w27:refnum<vi>)
  n153 = control-ref of="Timing Mode"() -> (w41:refnum<vi>)
  n154 = control-ref of="Slow Trigger Settings"() -> (w39:refnum<vi>)
  n155 = control-ref of="Phase Frontends"() -> (w28:refnum<vi>)
  n156 = control-ref of="Waiting Time"() -> (w54:refnum<vi>)
  n157 = control-ref of="Sequence length"() -> (w36:refnum<vi>)
  n158 = control-ref of="Seq SM State"() -> (w51:refnum<vi>)
  n159 = control-ref of="PSDB Shot Comment"() -> (w40:refnum<vi>)
  n160 = control-ref of="Experiment Description"() -> (w33:refnum<vi>)
  n161 = control-ref of="State PA Backreflection"() -> (w2:refnum<vi>)
  n162 = control-ref of="State PSDB"() -> (w1:refnum<vi>)
  n163 = control-ref of="State Timing"() -> (w3:refnum<vi>)
  n164 = control-ref of="Shottype"() -> (w35:refnum<vi>)
  n165 = control-ref of="Experiment"() -> (w34:refnum<vi>)
  n166 = control-ref of="PSDB Status"() -> (w62:refnum<vi>)
  n167 = call "PH_Class.Register Event.vi"("i ref in"="object ref", "error in (no error)"="error in (no error)") -> ("i ref out"=w67:refnum<vi>, "Event Registration Refnum"=w65:refnum<event-registration>, "error out"=w66:errorcluster)  [unwired: 15 in]
  n168 = while {
    tunnel: w67 -> [w252]
    tunnel: [w251] -> w187
    tunnel: [w254] -> w186
    tunnel: w66 -> [w253]
    tunnel: w65 -> [w250]
    tunnel: [w249] -> w64
    tunnel: w63 -> [w248]
    tunnel: w62 -> [w247]
    tunnel: w59 -> [w246]
    tunnel: w58 -> [w245]
    tunnel: w57 -> [w244]
    tunnel: w56 -> [w243]
    tunnel: w55 -> [w242]
    tunnel: w54 -> [w241]
    tunnel: w53 -> [w240]
    tunnel: w52 -> [w239]
    tunnel: w51 -> [w238]
    tunnel: w50 -> [w237]
    tunnel: w49 -> [w236]
    tunnel: w48 -> [w235]
    tunnel: w47 -> [w234]
    tunnel: w46 -> [w233]
    tunnel: w45 -> [w232]
    tunnel: w44 -> [w231]
    tunnel: w3 -> [w230]
    tunnel: w43 -> [w229]
    tunnel: w42 -> [w228]
    tunnel: w41 -> [w227]
    tunnel: w40 -> [w226]
    tunnel: w39 -> [w225]
    tunnel: w2 -> [w224]
    tunnel: w38 -> [w223]
    tunnel: w37 -> [w222]
    tunnel: w36 -> [w221]
    tunnel: w35 -> [w220]
    tunnel: w34 -> [w219]
    tunnel: w33 -> [w218]
    tunnel: w1 -> [w217]
    tunnel: w32 -> [w216]
    tunnel: w31 -> [w215]
    tunnel: w30 -> [w214]
    tunnel: w29 -> [w213]
    tunnel: w28 -> [w212]
    tunnel: w27 -> [w211]
    stop <- w255 stop-if-true
    n169 = event shown="[25] <Event>: User Event" {
      selector: w250 -> [_ _ _ _ _ _ _ _ _ _ _ _ _ _ _ _ _ _ _ _ _ _ _ _ _ _]
      dyn-events: [_ _ _ _ _ _ _ _ _ _ _ _ _ _ _ _ _ _ _ _ _ _ _ _ _ _] -> w249
      timeout: _ -> [_ _ _ _ _ _ _ _ _ _ _ _ _ _ _ _ _ _ _ _ _ _ _ _ _ _]
      tunnel: ["Delete" _ _ _ _ _ _ _ _ _ _ _ _ _ _ _ _ _ _ _ _ _ _ _ _ _] -> w255
      tunnel: w252 -> [w259 w263 w269 w275 w281 w286 w291 w298 w304 w310 w317 w325 w372 w408 w413 w418 w424 w428 w438 w456 w471 w490 w506 w513 w520 w567]
      tunnel: [w256 w264 w270 w276 w282 w287 w292 w295 w301 w307 w319 w327 w379 w409 w414 w419 w425 w429 w437 w453 w469 w480 w505 w508 w517 w526] -> w254
      tunnel: w253 -> [w258 w265 w271 w277 w283 w288 w293 w296 w302 w308 w315 w332 w381 w410 w415 w420 w426 w431 w440 w454 w470 w488 w503 w512 w523 w566]
      tunnel: [w257 w261 w267 w273 w279 w284 w289 w297 w303 w309 w318 w326 w380 w406 w411 w416 w421 w430 w435 w455 w468 w482 w504 w509 w519 w524] -> w251
      tunnel: w248 -> [_ _ _ _ _ _ _ _ _ _ _ _ _ _ _ _ _ _ _ _ _ _ _ _ _ w564]
      tunnel: w247 -> [_ _ _ _ _ _ _ _ _ _ _ _ _ _ _ _ _ _ _ _ _ _ _ _ _ w563]
      tunnel: w246 -> [_ _ _ _ _ _ _ _ _ _ _ _ _ _ _ _ _ _ _ _ _ _ _ _ _ w562]
      tunnel: w245 -> [_ _ _ _ _ _ _ _ _ _ _ _ _ _ _ _ _ _ _ _ _ _ _ _ _ w561]
      tunnel: w244 -> [_ _ _ _ _ _ _ _ _ _ _ _ _ _ _ _ _ _ _ _ _ _ _ _ _ w560]
      tunnel: w243 -> [_ _ _ _ _ _ _ _ _ _ _ _ _ _ _ _ _ _ _ _ _ _ _ _ _ w559]
      tunnel: w242 -> [_ _ _ _ _ _ _ _ _ _ _ _ _ _ _ _ _ _ _ _ _ _ _ _ _ w558]
      tunnel: w241 -> [_ _ _ _ _ _ _ _ _ _ _ _ _ _ _ _ _ _ _ _ _ _ _ _ _ w557]
      tunnel: w240 -> [_ _ _ _ _ _ _ _ _ _ _ _ _ _ _ _ _ _ _ _ _ _ _ _ _ w556]
      tunnel: w239 -> [_ _ _ _ _ _ _ _ _ _ _ _ _ _ _ _ _ _ _ _ _ _ _ _ _ w555]
      tunnel: w238 -> [_ _ _ _ _ _ _ _ _ _ _ _ _ _ _ _ _ _ _ _ _ _ _ _ _ w554]
      tunnel: w237 -> [_ _ _ _ _ _ _ _ _ _ _ _ _ _ _ _ _ _ _ _ _ _ _ _ _ w553]
      tunnel: w236 -> [_ _ _ _ _ _ _ _ _ _ _ _ _ _ _ _ _ _ _ _ _ _ _ _ _ w552]
      tunnel: w235 -> [_ _ _ _ _ _ _ _ _ _ _ _ _ _ _ _ _ _ _ _ _ _ _ _ _ w551]
      tunnel: w234 -> [_ _ _ _ _ _ _ _ _ _ _ _ _ _ _ _ _ _ _ _ _ _ _ _ _ w550]
      tunnel: w233 -> [_ _ _ _ _ _ _ _ _ _ _ _ _ _ _ _ _ _ _ _ _ _ _ _ _ w549]
      tunnel: w232 -> [_ _ _ _ _ _ _ _ _ _ _ _ _ _ _ _ _ _ _ _ _ _ _ _ _ w548]
      tunnel: w231 -> [_ _ _ _ _ _ _ _ _ _ _ _ _ _ _ _ _ _ _ _ _ _ _ _ _ w547]
      tunnel: w230 -> [_ _ _ _ _ _ _ _ _ _ _ _ _ _ _ _ _ _ _ _ _ _ _ _ _ w546]
      tunnel: w229 -> [_ _ _ _ _ _ _ _ _ _ _ _ _ _ _ _ _ _ _ _ _ _ _ _ _ w545]
      tunnel: w228 -> [_ _ _ _ _ _ _ _ _ _ _ _ _ _ _ _ _ _ _ _ _ _ _ _ _ w544]
      tunnel: w227 -> [_ _ _ _ _ _ _ _ _ _ _ _ _ _ _ _ _ _ _ _ _ _ _ _ _ w543]
      tunnel: w226 -> [_ _ _ _ _ _ _ _ _ _ _ _ _ _ _ _ _ _ _ _ _ _ _ _ _ w542]
      tunnel: w225 -> [_ _ _ _ _ _ _ _ _ _ _ _ _ _ _ _ _ _ _ _ _ _ _ _ _ w541]
      tunnel: w224 -> [_ _ _ _ _ _ _ _ _ _ _ _ _ _ _ _ _ _ _ _ _ _ _ _ _ w540]
      tunnel: w223 -> [_ _ _ _ _ _ _ _ _ _ _ _ _ _ _ _ _ _ _ _ _ _ _ _ _ w539]
      tunnel: w222 -> [_ _ _ _ _ _ _ _ _ _ _ _ _ _ _ _ _ _ _ _ _ _ _ _ _ w538]
      tunnel: w221 -> [_ _ _ _ _ _ _ _ _ _ _ _ _ _ _ _ _ _ _ _ _ _ _ _ _ w537]
      tunnel: w220 -> [_ _ _ _ _ _ _ _ _ _ _ _ _ _ _ _ _ _ _ _ _ _ _ _ _ w536]
      tunnel: w219 -> [_ _ _ _ _ _ _ _ _ _ _ _ _ _ _ _ _ _ _ _ _ _ _ _ _ w535]
      tunnel: w218 -> [_ _ _ _ _ _ _ _ _ _ _ _ _ _ _ _ _ _ _ _ _ _ _ _ _ w534]
      tunnel: w217 -> [_ _ _ _ _ _ _ _ _ _ _ _ _ _ _ _ _ _ _ _ _ _ _ _ _ w533]
      tunnel: w216 -> [_ _ _ _ _ _ _ _ _ _ _ _ _ _ _ _ _ _ _ _ _ _ _ _ _ w532]
      tunnel: w215 -> [_ _ _ _ _ _ _ _ _ _ _ _ _ _ _ _ _ _ _ _ _ _ _ _ _ w531]
      tunnel: w214 -> [_ _ _ _ _ _ _ _ _ _ _ _ _ _ _ _ _ _ _ _ _ _ _ _ _ w530]
      tunnel: w213 -> [_ _ _ _ _ _ _ _ _ _ _ _ _ _ _ _ _ _ _ _ _ _ _ _ _ w529]
      tunnel: w212 -> [_ _ _ _ _ _ _ _ _ _ _ _ _ _ _ _ _ _ _ _ _ _ _ _ _ w528]
      tunnel: w211 -> [_ _ _ _ _ _ _ _ _ _ _ _ _ _ _ _ _ _ _ _ _ _ _ _ _ w527]
      event "Delete": Value Change {
        n170 = event-data() -> ()  [unwired: 1 in, 1 out]
        n171 = call "PH_Class.Delete GUI.vi"("VI in"=w259, "error in (no error)"=w258) -> ("VI out"=w257:refnum<vi>, "error out"=w256:errorcluster)  [unwired: 16 in]
      }
      event "Main Off": Value Change {
        n172 = event-data() -> ()  [unwired: 1 in, 1 out]
        n173 = call "CSSystemLib.ref2name.vi"("obj refnum"=w263) -> ("name"=w262:string)
        n174 = call "PH_Sequencer.evt call Main Off.vi"("i ref in"=w263, "Instance"=w262, "error in (no error)"=w265) -> ("i ref out"=w261:refnum<vi>, "error out"=w264:errorcluster)  [unwired: 15 in]
      }
      event Value Change {
        n175 = event-data() -> ("NewVal"=w266:T4)  [unwired: 1 in]
        n176 = call "CSSystemLib.ref2name.vi"("obj refnum"=w269) -> ("name"=w268:string)
        n177 = call "PH_Sequencer.evt call set Timing Mode.vi"("i ref in"=w269, "Instance"=w268, "Timing Mode"=w266, "error in (no error)"=w271) -> ("i ref out"=w267:refnum<vi>, "error out"=w270:errorcluster)  [unwired: 14 in]
      }
      event Value Change {
        n178 = event-data() -> ("NewVal"=w272:T5)  [unwired: 1 in]
        n179 = call "CSSystemLib.ref2name.vi"("obj refnum"=w275) -> ("name"=w274:string)
        n180 = call "PH_Sequencer.evt call set Slow Trigger.vi"("i ref in"=w275, "Instance"=w274, "Slow Trigger Settings"=w272, "error in (no error)"=w277) -> ("i ref out"=w273:refnum<vi>, "error out"=w276:errorcluster)  [unwired: 14 in]
      }
      event Value Change {
        n181 = event-data() -> ("NewVal"=w278:T3)  [unwired: 1 in]
        n182 = call "CSSystemLib.ref2name.vi"("obj refnum"=w281) -> ("name"=w280:string)
        n183 = call "PH_Sequencer.evt call set Phase Frontends.vi"("i ref in"=w281, "Instance"=w280, "Phase FEs"=w278, "error in (no error)"=w283) -> ("i ref out"=w279:refnum<vi>, "error out"=w282:errorcluster)  [unwired: 14 in]
      }
      event "Get PSDB Info": Value Change {
        n184 = event-data() -> ()  [unwired: 1 in, 6 out]
        n185 = call "CSSystemLib.ref2name.vi"("obj refnum"=w286) -> ("name"=w285:string)
        n186 = call "PH_Sequencer.evt call get PSDB Info.vi"("i ref in"=w286, "Instance"=w285, "error in (no error)"=w288) -> ("i ref out"=w284:refnum<vi>, "error out"=w287:errorcluster)  [unwired: 15 in]
      }
      event "Set PSDB Settings": Value Change {
        n187 = event-data() -> ()  [unwired: 1 in, 6 out]
        n188 = call "CSSystemLib.ref2name.vi"("obj refnum"=w291) -> ("name"=w290:string)
        n189 = call "PH_Sequencer.evt call set PSDB Settings.vi"("i ref in"=w291, "Instance"=w290, "error in (no error)"=w293) -> ("i ref out"=w289:refnum<vi>, "error out"=w292:errorcluster)  [unwired: 15 in]
      }
      event "PSDB Shot Comment": Value Change {
        n190 = event-data() -> ("NewVal"=w294:string)  [unwired: 1 in]
        n191 = call "CSSystemLib.ref2name.vi"("obj refnum"=w298) -> ("name"=w299:string)
        n192 = call "PH_Sequencer.evt call Set Shot Comment.vi"("i ref in"=w298, "Instance"=w299, "Shot Comment"=w294, "error in (no error)"=w296) -> ("i ref out"=w297:refnum<vi>, "error out"=w295:errorcluster)  [unwired: 14 in]
      }
      event "Experiment": Value Change {
        n193 = event-data() -> ("NewVal"=w300:i16)  [unwired: 1 in]
        n194 = call "CSSystemLib.ref2name.vi"("obj refnum"=w304) -> ("name"=w305:string)
        n195 = call "PH_Sequencer.evt call Set Exp ID.vi"("i ref in"=w304, "Instance"=w305, "Experiment"=w300, "error in (no error)"=w302) -> ("i ref out"=w303:refnum<vi>, "error out"=w301:errorcluster)  [unwired: 14 in]
      }
      event "Shottype": Value Change {
        n196 = event-data() -> ("NewVal"=w306:i16)  [unwired: 1 in]
        n197 = call "CSSystemLib.ref2name.vi"("obj refnum"=w310) -> ("name"=w311:string)
        n198 = call "PH_Sequencer.evt call Set Shottype.vi"("i ref in"=w310, "Instance"=w311, "Shot Type"=w306, "error in (no error)"=w308) -> ("i ref out"=w309:refnum<vi>, "error out"=w307:errorcluster)  [unwired: 14 in]
      }
      event "Force Timing": Value Change {
        n199 = event-data() -> ()  [unwired: 1 in, 1 out]
        n200 = call "PH_Sequencer.get i attribute.vi"("i ref in"=w317, "error in (no error)"=w315) -> ("i ref out"=w316:refnum<vi>, "i attribute"=w313:T27, "error out"=w314:errorcluster)  [unwired: 15 in]
        n201 = Unbundle By Name(w313) -> ("Timing.Instance"=w312:string)
        n202 = call "PH_Timing.evt call ForceShot.vi"("i ref in"=w316, "Instance"=w312, "error in (no error)"=w314) -> ("i ref out"=w318:refnum<vi>, "error out"=w319:errorcluster)  [unwired: 15 in]
      }
      event "PPMA_PU1", "PPMA_PU2", "PPMA_PU3", "PPMA_PU4", "PPMA_PU5", "PPPA_19mm_1_PU", "PPPA_19mm_2_PU", "PPPA_45mm_MAIN_PU", "PPMA_FR", "PPPA_45mm_DP_PU": Value Change {
        n203 = event-data() -> ("CtlRef"=w330:refnum<vi>, "OldVal"=w331:bool, "NewVal"=w320:bool)  [unwired: 1 in]
        n204 = property class="Bool (strict)"(reference=w330, error in=w332, "Value"=w331) -> (error out=w324:errorcluster, "Label.Text"=w328:string)  [unwired: 1 out]
        n205 = call "CSSystemLib.ref2name.vi"("obj refnum"=w325) -> ("name"=w321:string)
        n206 = case shown="\"PPPA_45mm_MAIN_PU\"" w328 {
          tunnel: [PH_PP_Common.PUs."PA-19mm-1" ("Power Unit") PH_PP_Common.PUs."PA-19mm-2" ("Power Unit") PH_PP_Common.PUs."PA-45mm-MAIN" ("Power Unit") PH_PP_Common.PUs."MA-PU-1" ("Power Unit") PH_PP_Common.PUs."MA-PU-2" ("Power Unit") PH_PP_Common.PUs."MA-PU-3" ("Power Unit") PH_PP_Common.PUs."MA-PU-4" ("Power Unit") PH_PP_Common.PUs."MA-PU-5" ("Power Unit") PH_PP_Common.PUs."MA-FR" ("Power Unit") PH_PP_Common.PUs."PA-45mm-DP" ("Power Unit") PH_PP_Common.PUs."no Info" ("Power Unit")] -> w329
          tunnel: w325 -> [w334 w337 w345 w348 w351 w354 w357 w360 w363 w366 w369]
          tunnel: w324 -> [w333 w336 w343 w347 w350 w353 w356 w359 w362 w365 w368]
          tunnel: [w334 w337 w344 w348 w351 w354 w357 w360 w363 w366 w369] -> w323
          tunnel: [w333 w336 w342 w347 w350 w353 w356 w359 w362 w365 w368] -> w322
          tunnel: w321 -> [_ _ w340 _ _ _ _ _ _ _ _]
          tunnel: w320 -> [_ _ w339 _ _ _ _ _ _ _ _]
          frame "PPPA_19mm_1_PU" {
          }
          frame "PPPA_19mm_2_PU" {
          }
          frame "PPPA_45mm_MAIN_PU" {
            n207 = call "PH_Sequencer.evt call PP PU on.vi"("i ref in"=w345, "Sequencer Inst"=w340, "Power Unit"=PH_PP_Common.PUs."PA-45mm-PILC", "PP PU on"=w339, "error in (no error)"=w343) -> ("i ref out"=w344:refnum<vi>, "error out"=w342:errorcluster)  [unwired: 13 in]
          }
          frame "PPMA_PU1" {
          }
          frame "PPMA_PU2" {
          }
          frame "PPMA_PU3" {
          }
          frame "PPMA_PU4" {
          }
          frame "PPMA_PU5" {
          }
          frame "PPMA_FR" {
          }
          frame "PPPA_45mm_DP_PU" {
          }
          frame Default {
          }
        }
        n208 = call "PH_Sequencer.evt call PP PU on.vi"("i ref in"=w323, "Sequencer Inst"=w321, "Power Unit"=w329, "PP PU on"=w320, "error in (no error)"=w322) -> ("i ref out"=w326:refnum<vi>, "error out"=w327:errorcluster)  [unwired: 13 in]
      }
      event "Set Voltage PU 1", "Set Voltage PU 2", "Set Voltage PU 3", "Set Voltage PU 4", "Set Voltage PU 5", "Set Voltage PU 19mm - 1", "Set Voltage PU 19mm - 2", "Set Voltage PU 45mm", "Set Voltage FR", "Set Voltage PU 45mm DP": Value Change {
        n209 = event-data() -> ("CtlRef"=w376:refnum<vi>, "OldVal"=w377:dbl, "NewVal"=w378:dbl)  [unwired: 1 in]
        n210 = property class="DigNum (strict)"(reference=w376, error in=w381, "Value"=w377) -> (error out=w371:errorcluster, "Label.Text"=w375:string)  [unwired: 1 out]
        n211 = case shown="\"Set Voltage PU 45mm DP\"" w375 {
          tunnel: [PH_PP_Common.PUs."PA-19mm-1" ("Power Unit") PH_PP_Common.PUs."PA-19mm-2" ("Power Unit") PH_PP_Common.PUs."PA-45mm-MAIN" ("Power Unit") PH_PP_Common.PUs."MA-PU-1" ("Power Unit") PH_PP_Common.PUs."MA-PU-2" ("Power Unit") PH_PP_Common.PUs."MA-PU-3" ("Power Unit") PH_PP_Common.PUs."MA-PU-4" ("Power Unit") PH_PP_Common.PUs."MA-PU-5" ("Power Unit") PH_PP_Common.PUs."MA-FR" ("Power Unit") PH_PP_Common.PUs."PA-45mm-DP" ("Power Unit") w405] -> w374
          tunnel: [PH_PP_Common.PUs."no Info" ("Power Unit") PH_PP_Common.PUs."no Info" ("Power Unit") PH_PP_Common.PUs."PA-45mm-PILC" ("Power Unit") PH_PP_Common.PUs."no Info" ("Power Unit") PH_PP_Common.PUs."no Info" ("Power Unit") PH_PP_Common.PUs."no Info" ("Power Unit") PH_PP_Common.PUs."no Info" ("Power Unit") PH_PP_Common.PUs."no Info" ("Power Unit") PH_PP_Common.PUs."no Info" ("Power Unit") PH_PP_Common.PUs."no Info" ("Power Unit") w405] -> w373
          frame "Set Voltage PU 19mm - 1" {
          }
          frame "Set Voltage PU 19mm - 2" {
          }
          frame "Set Voltage PU 45mm" {
          }
          frame "Set Voltage PU 1" {
          }
          frame "Set Voltage PU 2" {
          }
          frame "Set Voltage PU 3" {
          }
          frame "Set Voltage PU 4" {
          }
          frame "Set Voltage PU 5" {
          }
          frame "Set Voltage FR" {
          }
          frame "Set Voltage PU 45mm DP" {
          }
          frame Default {
            w405 = PH_PP_Common.PUs."no Info" ("Power Unit")
          }
        }
        n212 = call "CSSystemLib.ref2name.vi"("obj refnum"=w372) -> ("name"=w382:string)
        n213 = call "PH_Sequencer.evt call SetPPVoltage.vi"("i ref in"=w372, "Sequencer Inst"=w382, "Power Unit"=w374, "PP Voltage [V]"=w378, "error in (no error)"=w371) -> ("i ref out"=w384:refnum<vi>, "error out"=w383:errorcluster)  [unwired: 13 in]
        n214 = call "PH_Sequencer.evt call SetPPVoltage.vi"("i ref in"=w384, "Sequencer Inst"=w382, "Power Unit"=w373, "PP Voltage [V]"=w378, "error in (no error)"=w383) -> ("i ref out"=w380:refnum<vi>, "error out"=w379:errorcluster)  [unwired: 13 in]
      }
      event "Fire": Mouse Up {
        n215 = event-data() -> ()  [unwired: 1 in, 1 out]
        n216 = call "CSSystemLib.ref2name.vi"("obj refnum"=w408) -> ("name"=w407:string)
        n217 = call "PH_Sequencer.evt call Shot.vi"("i ref in"=w408, "Sequencer Instance"=w407, "error in (no error)"=w410) -> ("i ref out"=w406:refnum<vi>, "error out"=w409:errorcluster)  [unwired: 15 in]
      }
      event "Clear Beamline": Value Change {
        n218 = event-data() -> ()  [unwired: 1 in, 1 out]
        n219 = call "CSSystemLib.ref2name.vi"("obj refnum"=w413) -> ("name"=w412:string)
        n220 = call "PH_Sequencer.evt call Clear Beamline.vi"("i ref in"=w413, "Instance"=w412, "error in (no error)"=w415) -> ("i ref out"=w411:refnum<vi>, "error out"=w414:errorcluster)  [unwired: 15 in]
      }
      event "Clear Z6 Beamline": Value Change {
        n221 = event-data() -> ()  [unwired: 1 in, 1 out]
        n222 = call "CSSystemLib.ref2name.vi"("obj refnum"=w418) -> ("name"=w417:string)
        n223 = call "PH_Sequencer.evt call Clear Z6 Beamline.vi"("i ref in"=w418, "Instance"=w417, "error in (no error)"=w420) -> ("i ref out"=w416:refnum<vi>, "error out"=w419:errorcluster)  [unwired: 15 in]
      }
      event "Calorimeter": Value Change {
        n224 = event-data() -> ()  [unwired: 1 in, 1 out]
        n225 = call "CSSystemLib.ref2name.vi"("obj refnum"=w424) -> ("name"=w423:string)
        n226 = call "PH_Sequencer.evt call Set Calorimeter.vi"("i ref in"=w424, "Instance"=w423, "Calorimeter On"="Calorimeter", "error in (no error)"=w426) -> ("i ref out"=w421:refnum<vi>, "error out"=w425:errorcluster)  [unwired: 14 in]
      }
      event "Take Snapshot": Value Change {
        n227 = event-data() -> ()  [unwired: 1 in, 1 out]
        n228 = call "CSSystemLib.ref2name.vi"("obj refnum"=w428) -> ("name"=w427:string)
        n229 = call "PH_Sequencer.evt call get Snapshot.vi"("i ref in"=w428, "Instance"=w427, "error in (no error)"=w431) -> ("i ref out"=w430:refnum<vi>, "error out"=w429:errorcluster)  [unwired: 15 in]
      }
      event "Remember": Value Change {
        n230 = event-data() -> ()  [unwired: 1 in, 1 out]
        n231 = call "PH_Sequencer.get data to modify.vi"("i ref in"=w438, "error in (no error)"=w440) -> ("i ref out"=w436:refnum<vi>, "i attribute"=w433:T27, "timed out"=w434:bool, "error out"=w439:errorcluster)  [unwired: 14 in]
        n232 = case shown="False" w434 {
          tunnel: w439 -> [w447 w448]
          tunnel: [w446 w448] -> w437
          tunnel: w436 -> [w445 w449]
          tunnel: [w444 w449] -> w435
          tunnel: w433 -> [w443 _]
          tunnel: "Remember" -> [w441 _]
          frame False {
            n233 = Bundle By Name(cluster=w443, "PSDB.Remember Settings"=w441) -> (w442:T27)
            n234 = call "PH_Sequencer.set modified data.vi"("i ref in"=w445, "i attribute"=w442, "error in (no error)"=w447) -> ("i ref out"=w444:refnum<vi>, "error out"=w446:errorcluster)  [unwired: 15 in]
          }
          frame True {
          }
        }
      }
      event "Source YLF", "Source fs-Frontend", "Source ns-Frontend": Value Change {
        n235 = event-data() -> ("CtlRef"=w451:refnum<vi>, "OldVal"=w450:bool, "NewVal"=w452:bool)  [unwired: 1 in]
        n236 = property class="Bool (strict)"(reference=w451, error in=w454, "Value"=w450) -> (error out=w460:errorcluster, "Label.Text"=w458:string)  [unwired: 1 out]
        n237 = case shown="\"Source ns-Frontend\"" w458 {
          tunnel: [PH_BeamlineController.Sources."None" ("Source") PH_BeamlineController.Sources."YLF" ("Source") PH_BeamlineController.Sources."fs-Frontend" ("Source") PH_BeamlineController.Sources."ns-Frontend" ("Source")] -> w459
          frame Default {
          }
          frame "Source YLF" {
          }
          frame "Source fs-Frontend" {
          }
          frame "Source ns-Frontend" {
          }
        }
        n238 = call "CSSystemLib.ref2name.vi"("obj refnum"=w456) -> ("name"=w457:string)
        n239 = call "PH_BeamlineController.Event Call Select Source.vi"("i ref in"=w456, "Instance"=w457, "Source"=w459, "on(off"=w452, "error in (no error)"=w460) -> ("i ref out"=w455:refnum<vi>, "error out"=w453:errorcluster)  [unwired: 13 in]
      }
      event "Dump PA Delayed", "Dump PA Undelayed": Value Change {
        n240 = event-data() -> ("CtlRef"=w465:refnum<vi>, "OldVal"=w466:bool, "NewVal"=w467:bool)  [unwired: 1 in]
        n241 = property class="Bool (strict)"(reference=w465, error in=w470, "Value"=w466) -> (error out=w475:errorcluster, "Label.Text"=w473:string)  [unwired: 1 out]
        n242 = case shown="\"Dump PA Delayed\"" w473 {
          tunnel: [PH_BeamlineController.PA_DP_Targets."None" ("Targets") PH_BeamlineController.PA_DP_Targets."Dump PA Delayed Beam" ("Targets") PH_BeamlineController.PA_DP_Targets."Dump PA Undelayed Beam" ("Targets")] -> w474
          frame Default {
          }
          frame "Dump PA Delayed" {
          }
          frame "Dump PA Undelayed" {
          }
        }
        n243 = call "CSSystemLib.ref2name.vi"("obj refnum"=w471) -> ("name"=w472:string)
        n244 = call "PH_BeamlineController.Event Call Select PA DP Target.vi"("i ref in"=w471, "Instance"=w472, "PA DP Targets"=w474, "on(off"=w467, "error in (no error)"=w475) -> ("i ref out"=w468:refnum<vi>, "error out"=w469:errorcluster)  [unwired: 13 in]
      }
      event "Target PreAmp", "Target Calorimeter", "Target Dump Laserlabor", "Target Exp Laserlabor", "Target Dump Laserbay", "Target Exp Laserbay", "Target Dump Z6", "Target Exp Z6": Value Change {
        n245 = event-data() -> ("CtlRef"=w487:refnum<vi>, "OldVal"=w486:bool, "NewVal"=w489:bool)  [unwired: 1 in]
        n246 = property class="Bool (strict)"(reference=w487, error in=w488, "Value"=w486) -> (error out=w493:errorcluster, "Label.Text"=w491:string)  [unwired: 1 out]
        n247 = case shown="\"Target PreAmp\"" w491 {
          tunnel: [PH_BeamlineController.Targets."None" ("Targets") PH_BeamlineController.Targets."PreAmp" ("Targets") PH_BeamlineController.Targets."Dump Exp Laserlab" ("Targets") PH_BeamlineController.Targets."Exp Laserlab" ("Targets") PH_BeamlineController.Targets."Calorimeter" ("Targets") PH_BeamlineController.Targets."Dump Exp Laserbay" ("Targets") PH_BeamlineController.Targets."Exp Laserbay" ("Targets") PH_BeamlineController.Targets."Dump Exp Z6" ("Targets") PH_BeamlineController.Targets."Exp Z6" ("Targets")] -> w492
          frame Default {
          }
          frame "Target PreAmp" {
          }
          frame "Target Dump Laserlabor" {
          }
          frame "Target Exp Laserlabor" {
          }
          frame "Target Calorimeter" {
          }
          frame "Target Dump Laserbay" {
          }
          frame "Target Exp Laserbay" {
          }
          frame "Target Dump Z6" {
          }
          frame "Target Exp Z6" {
          }
        }
        n248 = call "CSSystemLib.ref2name.vi"("obj refnum"=w490) -> ("name"=w479:string)
        n249 = call "PH_BeamlineController.Event Call Select Target.vi"("i ref in"=w490, "Instance"=w479, "Targets"=w492, "on(off"=w489, "error in (no error)"=w493) -> ("i ref out"=w484:refnum<vi>, "error out"=w485:errorcluster)  [unwired: 13 in]
        n250 = call "PH_Sequencer.evt call Clear Beamline.vi"("i ref in"=w484, "Instance"=w479, "error in (no error)"=w485) -> ("i ref out"=w483:refnum<vi>, "error out"=w481:errorcluster)  [unwired: 15 in]
        n251 = call "PH_Sequencer.evt call Clear Z6 Beamline.vi"("i ref in"=w483, "Instance"=w479, "error in (no error)"=w481) -> ("i ref out"=w482:refnum<vi>, "error out"=w480:errorcluster)  [unwired: 15 in]
      }
      event "Accept current Path": Value Change {
        n252 = event-data() -> ()  [unwired: 1 in, 1 out]
        n253 = call "CSSystemLib.ref2name.vi"("obj refnum"=w506) -> ("name"=w507:string)
        n254 = call "PH_BeamlineController.Event Call Accept.vi"("i ref in"=w506, "Instance"=w507, "error in (no error)"=w503) -> ("i ref out"=w504:refnum<vi>, "error out"=w505:errorcluster)  [unwired: 15 in]
      }
      event "fs_Synchrolock_Watch": Value Change {
        n255 = event-data() -> ("CtlRef"=w511:refnum<vi>, "OldVal"=w510:bool)  [unwired: 1 in]
        n256 = property class="Bool (strict)"(reference=w511, error in=w512, "Value"=w510) -> (error out=w515:errorcluster)  [unwired: 1 out]
        n257 = call "PH_Synchrolock_Watch.evt call Reset Mira Warning.vi"("i ref in"=w513, "Instance"="fs_Synchrolock_Watch" ("Synchrolock.Instance"), "error in (no error)"=w515) -> ("i ref out"=w509:refnum<vi>, "error out"=w508:errorcluster)  [unwired: 15 in]
      }
      event "PA-Backreflection-Meas": Value Change {
        n258 = event-data() -> ("CtlRef"=w522:refnum<vi>, "OldVal"=w521:bool)  [unwired: 1 in]
        n259 = property class="Bool (strict)"(reference=w522, error in=w523, "Value"=w521) -> (error out=w518:errorcluster)  [unwired: 1 out]
        n260 = call "PH_BackreflectionMeas.evt call Reset Warning.vi"("i ref in"=w520, "Instance"="PA-Backreflection-Meas" ("Instance PA Backreflection"), "error in (no error)"=w518) -> ("i ref out"=w519:refnum<vi>, "error out"=w517:errorcluster)  [unwired: 15 in]
      }
      event User Event {
        n261 = event-data() -> ("Class"=w568:string)  [unwired: 1 in]
        n262 = case shown="\"PH_Sequencer\"" w568 {
          selector: w568 -> [_ w616]
          tunnel: w567 -> [w610 w624]
          tunnel: [w570 w620] -> w525
          tunnel: w566 -> [w609 w623]
          tunnel: [w569 w618] -> w565
          tunnel: w564 -> [_ w622]
          tunnel: w563 -> [_ w617]
          tunnel: w562 -> [w606 _]
          tunnel: w561 -> [w605 _]
          tunnel: w560 -> [w604 _]
          tunnel: w559 -> [w603 _]
          tunnel: w558 -> [w602 _]
          tunnel: w557 -> [w601 _]
          tunnel: w556 -> [w600 _]
          tunnel: w555 -> [w599 _]
          tunnel: w554 -> [w598 _]
          tunnel: w553 -> [w597 _]
          tunnel: w552 -> [w596 _]
          tunnel: w551 -> [w595 _]
          tunnel: w550 -> [w594 _]
          tunnel: w549 -> [w593 _]
          tunnel: w548 -> [w592 _]
          tunnel: w547 -> [w591 _]
          tunnel: w546 -> [w590 _]
          tunnel: w545 -> [w589 _]
          tunnel: w544 -> [w588 _]
          tunnel: w543 -> [w587 _]
          tunnel: w542 -> [w586 _]
          tunnel: w541 -> [w585 _]
          tunnel: w540 -> [w584 _]
          tunnel: w539 -> [w583 _]
          tunnel: w538 -> [w582 _]
          tunnel: w537 -> [w581 _]
          tunnel: w536 -> [w580 _]
          tunnel: w535 -> [w579 _]
          tunnel: w534 -> [w578 _]
          tunnel: w533 -> [w577 _]
          tunnel: w532 -> [w576 _]
          tunnel: w531 -> [w575 _]
          tunnel: w530 -> [w574 _]
          tunnel: w529 -> [w573 _]
          tunnel: w528 -> [w572 _]
          tunnel: w527 -> [w571 _]
          frame "PH_Sequencer" {
            n263 = call "PH_Sequencer.get data to modify.vi"("i ref in"=w610, "ms timeout (10000)"=-1, "error in (no error)"=w609) -> ("i ref out"=w613:refnum<vi>, "i attribute"=w611:T27, "error out"=w615:errorcluster)  [unwired: 13 in, 1 out]
            n264 = Bundle By Name(cluster=w611, "PUs"=w606, "GUI Refs.Main Off"=w605, "GUI Refs.Fire"=w604, "GUI Refs.Status"=w603, "GUI Refs.Ready"=w602, "GUI Refs.Waiting Time"=w601, "GUI Refs.Timeout"=w600, "GUI Refs.PPMA Ready"=w599, "GUI Refs.Sequencer SM State"=w598, "GUI Refs.PPPA Ready"=w597, "GUI Refs.Calorimeter"=w596, "GUI Refs.Beamline Ready"=w595, "GUI Refs.Clear Beamline"=w594, "GUI Refs.Linkage PPMA Rods"=w593, "GUI Refs.Linkage Current PA"=w592, "GUI Refs.Linkage Current MA"=w591, "GUI Refs.State Timing"=w590, "GUI Refs.Timing Ready"=w589, "GUI Refs.Force Timing"=w588, "GUI Refs.Timing Mode"=w587, "GUI Refs.PSDB Shot Comment"=w586, "GUI Refs.Slow Trigger Settings"=w585, "GUI Refs.State PA Backreflection"=w584, "GUI Refs.Beamline Z6 Ready"=w583, "GUI Refs.Clear Z6 Beamline"=w582, "GUI Refs.Sequence length"=w581, "GUI Refs.Shottype"=w580, "GUI Refs.Experiment"=w579, "GUI Refs.Experiment Description"=w578, "GUI Refs.State PSDB"=w577, "GUI Refs.PSDB Ready"=w576, "GUI Refs.Set PSDB Settings"=w575, "GUI Refs.Get PSDB Info"=w574, "GUI Refs.Take Snapshot"=w573, "GUI Refs.Phase Frontends"=w572, "GUI Refs.PP 45mm PILC in use"=w571) -> (w612:T27)
            n265 = call "PH_Sequencer.set modified data.vi"("i ref in"=w613, "i attribute"=w612, "error in (no error)"=w615) -> ("i ref out"=w608:refnum<vi>, "error out"=w607:errorcluster)  [unwired: 15 in]
            n266 = call "PH_Sequencer.set GUI elements to default.vi"("i ref in"=w608, "error in (no error)"=w607) -> ("i ref out"=w570:refnum<vi>, "error out"=w569:errorcluster)  [unwired: 16 in]
          }
          frame Default {
            n267 = call "PH_BeamlineController.set GUI Refs.vi"("Ref in"=w624, "Class"=w616, "Beamline Controller GUI Refs"=w622, "error in"=w623) -> ("Ref out"=w621:refnum<vi>, "error out"=w619:errorcluster)  [unwired: 14 in]
            n268 = call "PH_PSDBWriter.set GUI Refs.vi"("i ref in"=w621, "Class"=w616, "Ref PSDB Status"=w617, "error in"=w619) -> ("i ref out"=w620:refnum<vi>, "error out"=w618:errorcluster)  [unwired: 14 in]
          }
        }
        n269 = call "PH_Class.set GUI Refs stored Occurence.vi"("i ref in"=w525, "error in (no error)"=w565) -> ("i ref out"=w524:refnum<vi>, "error out"=w526:errorcluster)  [unwired: 16 in]
      }
    }
  }
  "error out" <- w186
  n270 = property on="Slow Trigger Settings" class="Clust (strict)"("Disabled"=u8 0) -> ()  [unwired: 2 in, 2 out]
  n271 = call "PH_Interaction.Super Destroy Me.vi"("i ref out"=w187) -> ()
  n272 = Unregister For Events(event registration refnum=w64) -> ()  [unwired: 1 in, 1 out]
